vi "数据表比对.vi"(8 "error in (no error)":errorcluster, 9 "查询元素输入":string(combo), 10 "仪器日志参数":string, 11 "table输入":string(combo)) -> (0 "error out":errorcluster, 1 "columns输出":string[](array[string]), 2 "待发送第一条数据":string[](array[string]), 3 "待发送数据":string[][](table))   [LabVIEW 2016, in "数据传输系统.lvlib"]
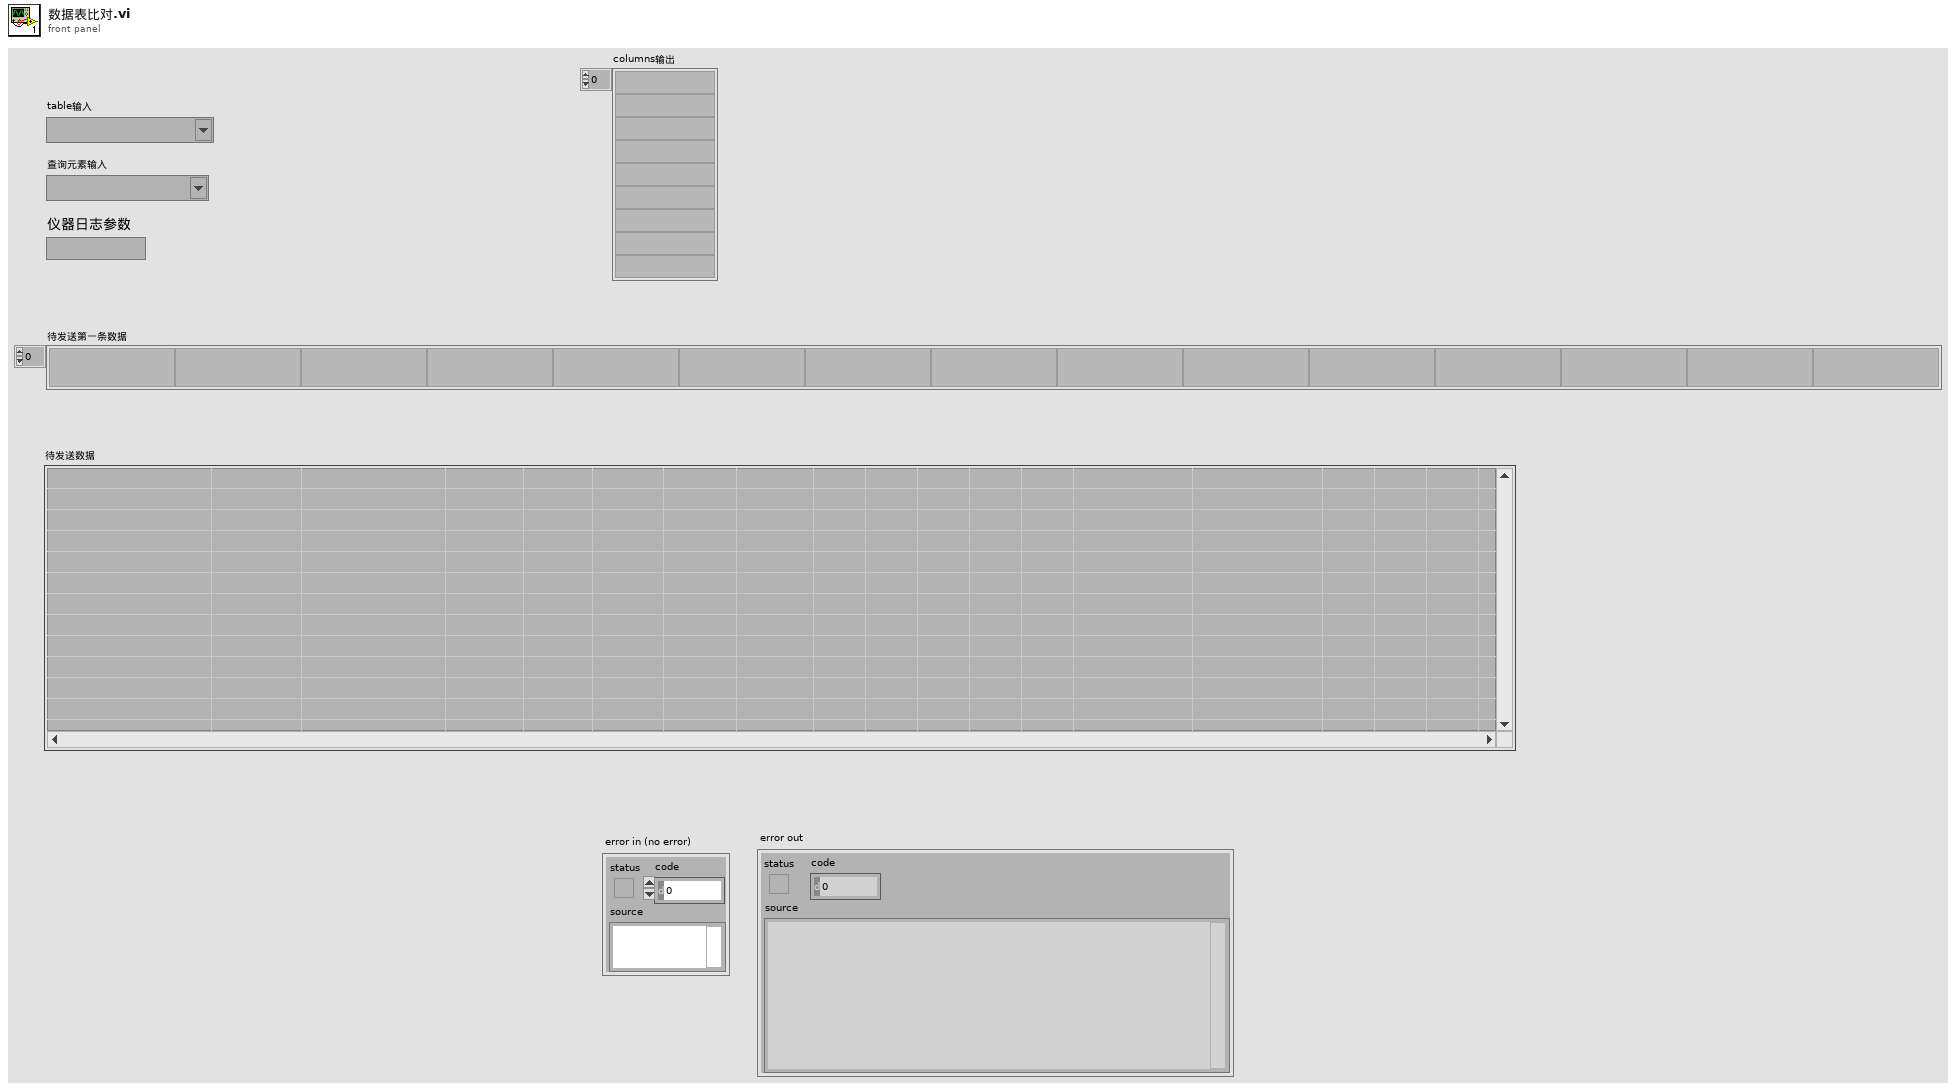
[diagram p1: front panel]
types:
  T1 = cluster{"氨氮仪器日志索引起始时间":string, "总磷仪器日志索引起始时间":string, "总氮仪器日志索引起始时间":string, "CODMn仪器日志索引起始时间":string, "CODCr仪器日志索引起始时间":string, "系统仪器日志索引起始时间":string, "氟化物仪器日志索引起始时间":string, "挥发酚仪器日志索引起始时间":string}
  T2 = cluster{"氨氮仪器参数索引起始时间":string, "总磷仪器参数索引起始时间":string, "总氮仪器参数索引起始时间":string, "CODMn仪器参数索引起始时间":string, "CODCr仪器参数索引起始时间":string, "DO仪器参数索引起始时间":string, "PH仪器参数索引起始时间":string, "比电导率仪器参数索引起始时间":string, "水温仪器参数索引起始时间":string, "浊度仪器参数索引起始时间":string, "叶绿素a仪器参数索引起始时间":string, "藻密度仪器参数索引起始时间":string, "ORP仪器参数索引起始时间":string, "氟化物仪器参数索引起始时间":string, "挥发酚仪器参数索引起始时间":string}
  T3 = typedef "数据传输系统.lvlib/应用环境.ctl" = enum16{"STD", "GB212", "婉仪平台"}
  T4 = cluster{"氨氮报警信息索引起始时间":string, "总磷报警信息索引起始时间":string, "总氮报警信息索引起始时间":string, "CODMn报警信息索引起始时间":string, "CODCr报警信息索引起始时间":string, "DO报警信息索引起始时间":string, "PH报警信息索引起始时间":string, "比电导率报警信息索引起始时间":string, "水温报警信息索引起始时间":string, "浊度报警信息索引起始时间":string, "叶绿素报警信息索引起始时间":string, "系统报警信息索引起始时间":string, "氟化物报警信息索引起始时间":string, "挥发酚报警信息索引起始时间":string}
  T5 = cluster{"氨氮零点核查索引起始时间":string, "总磷零点核查索引起始时间":string, "总氮零点核查索引起始时间":string, "CODMn零点核查索引起始时间":string, "CODCr零点核查索引起始时间":string, "亚硝酸盐零点核查索引起始时间":string, "硫化物零点核查索引起始时间":string, "ORP零点核查索引起始时间":string, "氟化物零点核查索引起始时间":string, "挥发酚零点核查索引起始时间":string}
  T6 = cluster{"氨氮标样核查索引起始时间":string, "总磷标样核查索引起始时间":string, "总氮标样核查索引起始时间":string, "CODMn标样核查索引起始时间":string, "CODCr标样核查索引起始时间":string, "DO标样核查索引起始时间":string, "PH标样核查索引起始时间":string, "比电导率标样核查索引起始时间":string, "水温标样核查索引起始时间":string, "浊度标样核查索引起始时间":string, "叶绿素a标样核查索引起始时间":string, "藻密度标样核查索引起始时间":string, "亚硝酸盐标样核查索引起始时间":string, "硫化物标样核查索引起始时间":string, "ORP标样核查索引起始时间":string, "氟化物标样核查索引起始时间":string, "挥发酚标样核查索引起始时间":string, "氯化物标样核查索引起始时间":string}
  T7 = cluster{"氨氮跨度核查索引起始时间":string, "总磷跨度核查索引起始时间":string, "总氮跨度核查索引起始时间":string, "CODMn跨度核查索引起始时间":string, "CODCr跨度核查索引起始时间":string, "亚硝酸盐跨度核查索引起始时间":string, "硫化物跨度核查索引起始时间":string, "ORP跨度核查索引起始时间":string, "氟化物跨度核查索引起始时间":string, "挥发酚跨度核查索引起始时间":string}
  T8 = typedef "LVDateTimeRec.ctl" = cluster{"秒数的小数部分":dbl, "秒":i32, "分":i32, "时":i32, "日":i32, "月":i32, "年":i32, "天数（周）":i32, "天数（年）":i32, "DST":i32}
  T9 = cluster{"氨氮加标回收索引起始时间":string, "总磷加标回收索引起始时间":string, "总氮加标回收索引起始时间":string, "CODMn加标回收索引起始时间":string, "CODCr加标回收索引起始时间":string, "氟化物加标回收索引起始时间":string, "挥发酚加标回收索引起始时间":string}
  T10 = cluster{"氨氮平行样索引起始时间":string, "总磷平行样索引起始时间":string, "总氮平行样索引起始时间":string, "CODMn平行样索引起始时间":string, "CODCr平行样索引起始时间":string, "氟化物平行样索引起始时间":string, "挥发酚平行样索引起始时间":string}
  T11 = cluster{"氨氮集成干预索引起始时间":string, "总磷集成干预索引起始时间":string, "总氮集成干预索引起始时间":string, "CODMn集成干预索引起始时间":string, "CODCr集成干预索引起始时间":string, "DO集成干预索引起始时间":string, "PH集成干预索引起始时间":string, "比电导率集成干预索引起始时间":string, "水温集成干预索引起始时间":string, "浊度集成干预索引起始时间":string, "叶绿素a集成干预索引起始时间":string, "藻密度集成干预索引起始时间":string, "亚硝酸盐集成干预索引起始时间":string, "硫化物集成干预索引起始时间":string, "ORP集成干预索引起始时间":string, "氟化物集成干预索引起始时间":string, "挥发酚集成干预索引起始时间":string, "氯化物集成干预索引起始时间":string}
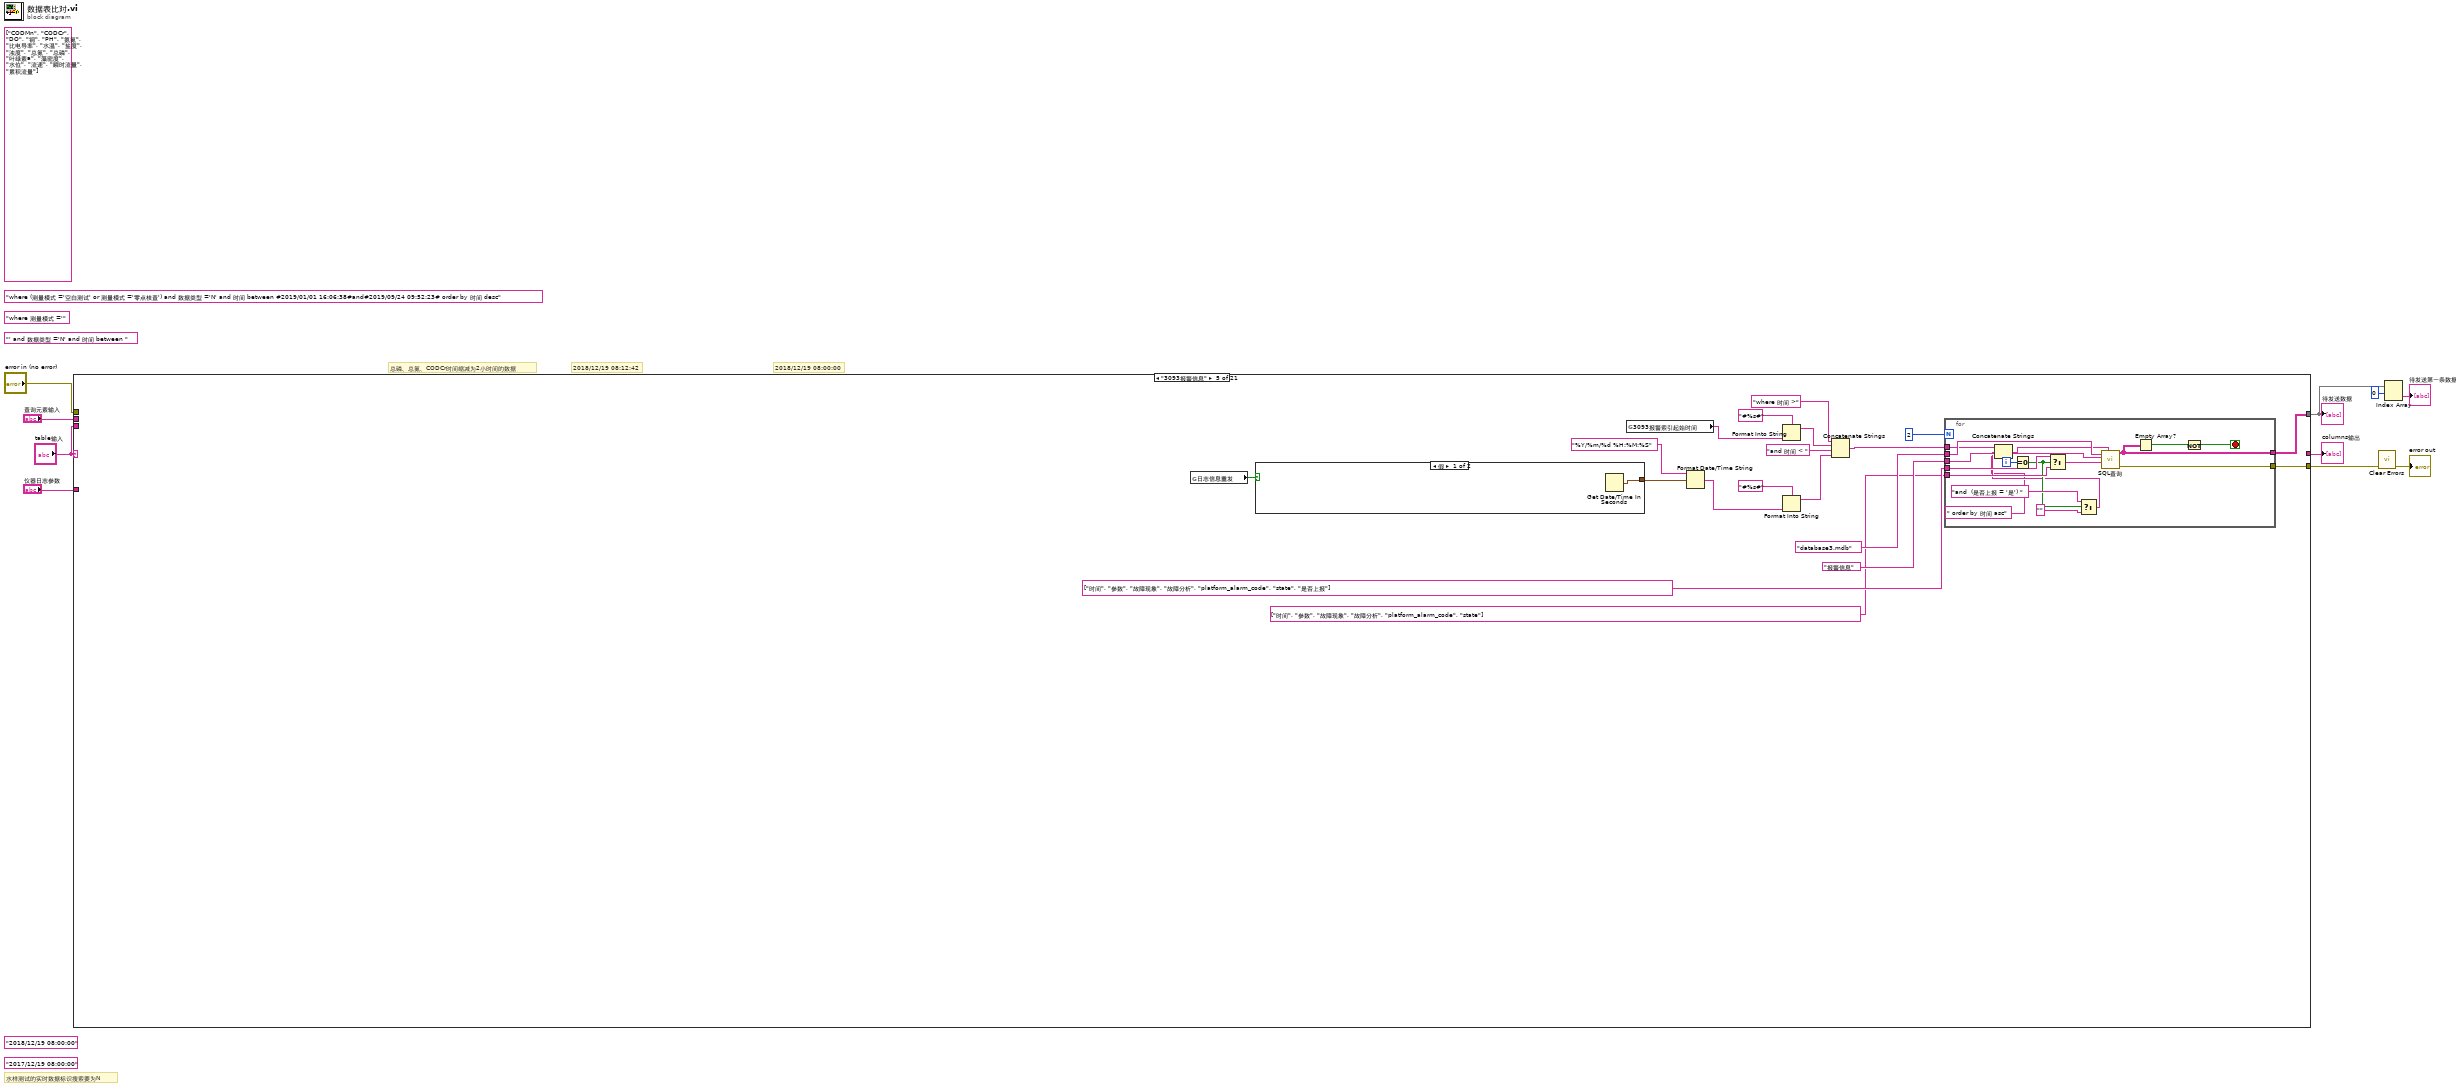
[diagram p0: block diagram]
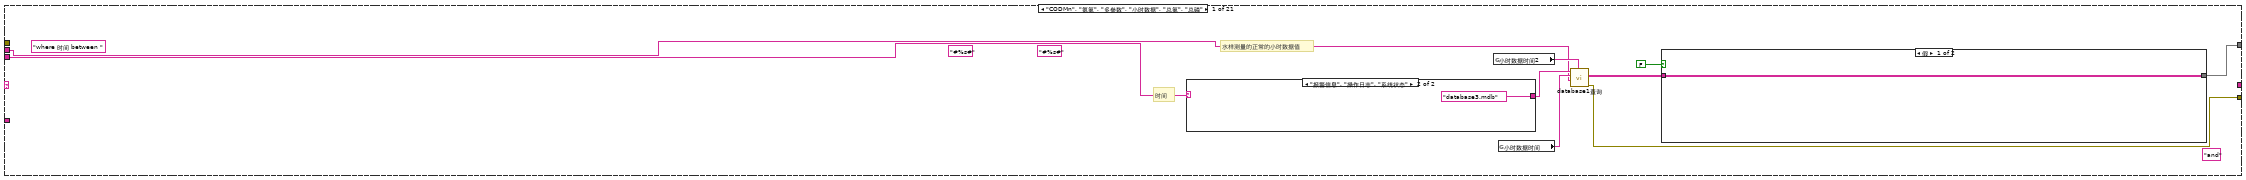
[diagram p2: hidden frame]
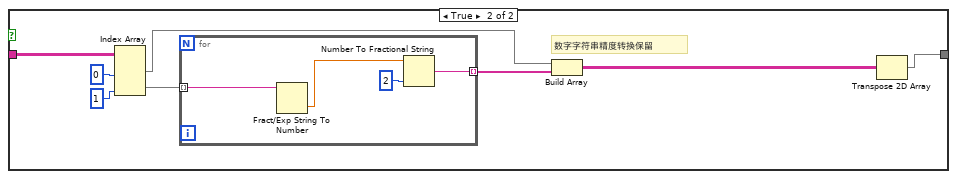
[diagram p3: hidden frame]
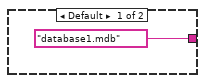
[diagram p4: hidden frame]
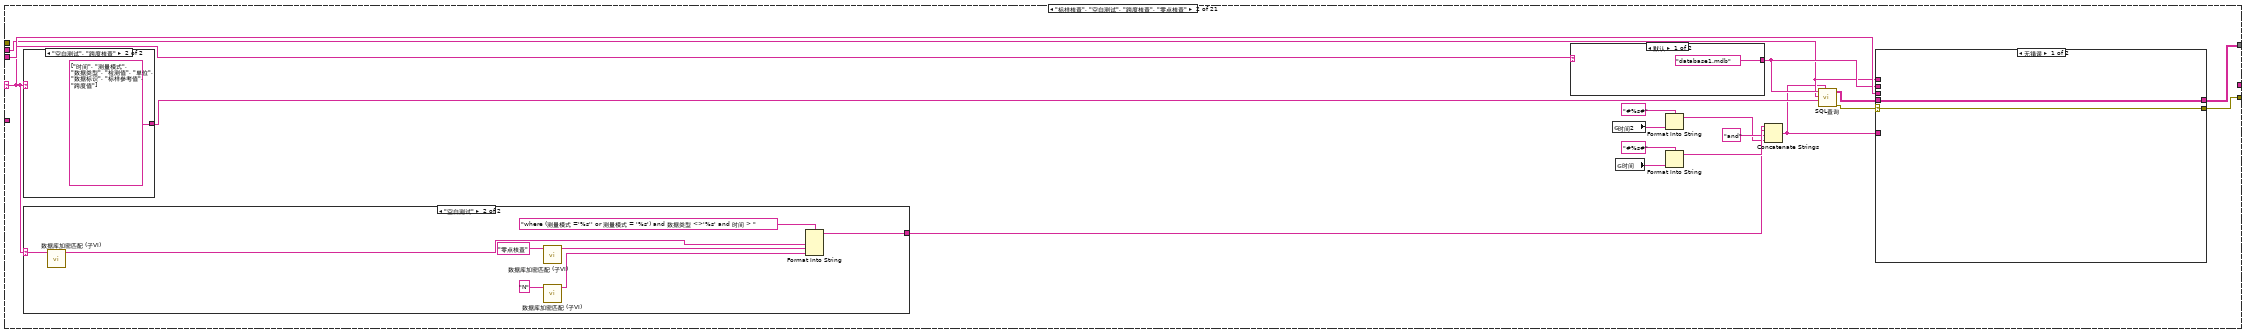
[diagram p5: hidden frame]
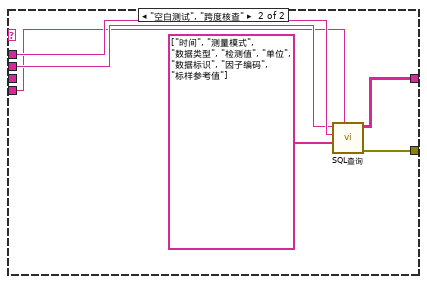
[diagram p7: hidden frame]
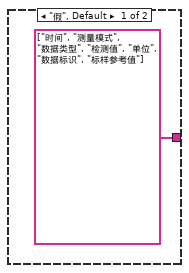
[diagram p8: hidden frame]
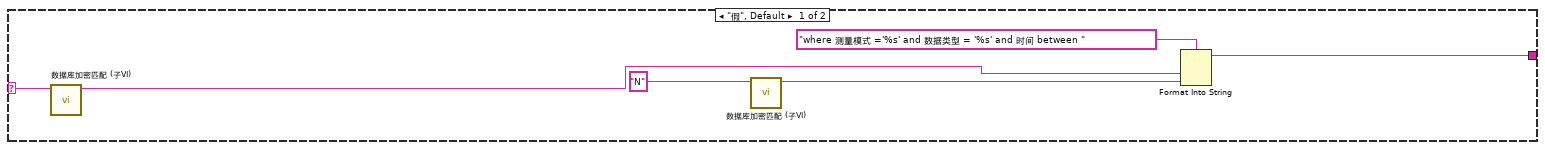
[diagram p9: hidden frame]
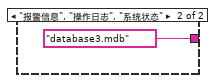
[diagram p10: hidden frame]
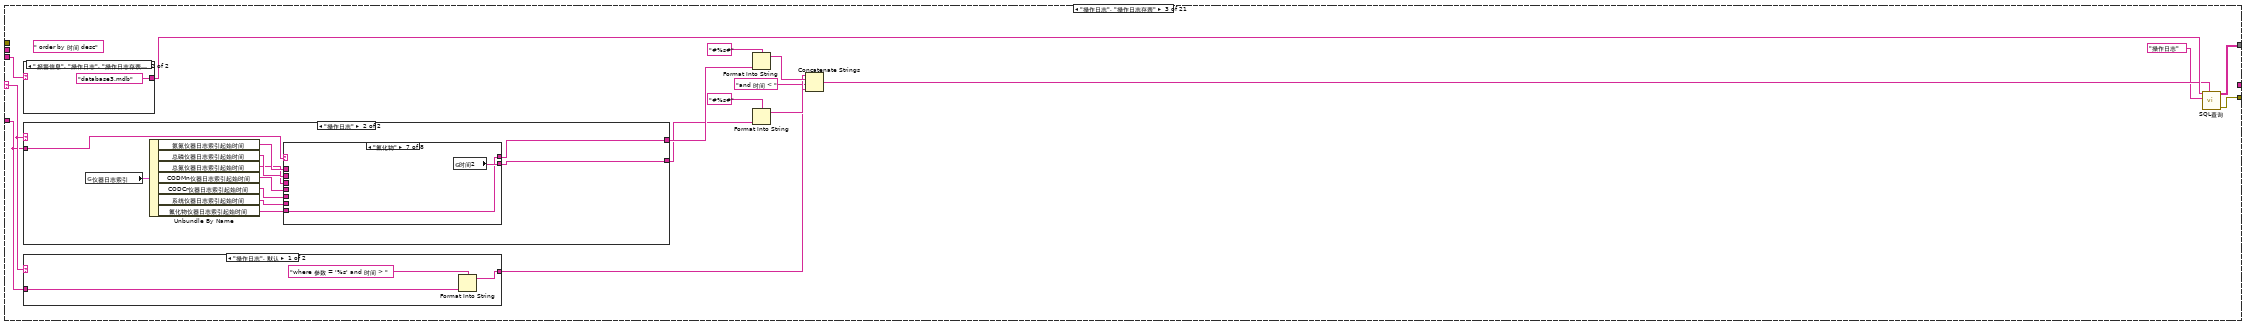
[diagram p11: hidden frame]
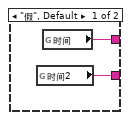
[diagram p12: hidden frame]
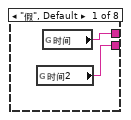
[diagram p13: hidden frame]
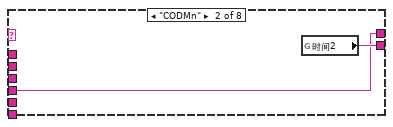
[diagram p14: hidden frame]
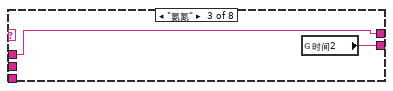
[diagram p15: hidden frame]
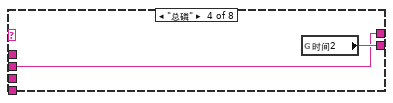
[diagram p16: hidden frame]
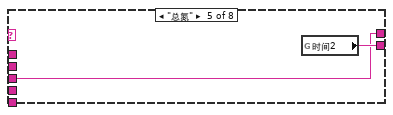
[diagram p17: hidden frame]
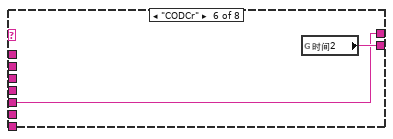
[diagram p18: hidden frame]
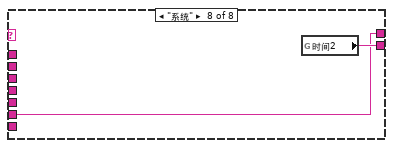
[diagram p19: hidden frame]
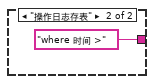
[diagram p20: hidden frame]
diagram:
  (unwired) "' and 数据类型 ='N' and 时间 between "
  (unwired) "where 测量模式 ='" ("condition")
  (unwired) "where (测量模式 ='空白测试' or 测量模式 ='零点核查') and 数据类型 ='N' and 时间 between #2019/01/01 16:06:38#and#2019/09/24 09:52:23# order by 时间 desc" ("condition")
  (unwired) string[] ["CODMn", "CODCr", "DO", "铜", "PH", "氨氮", "比电导率", "水温", "盐度", "浊度", "总氮", "总磷", "叶绿素a", "藻密度", "水位", "流速", "瞬时流量", "累积流量"] ("查询参数数组")
  (unwired) "2017/12/19 08:00:00"
  (unwired) "2018/12/19 08:00:00"
  # "水样测试的实时数据标识搜索要为N"
  # "2018/12/19 08:00:00"
  # "总磷、总氮、CODCr时间缩减为2小时间的数据"
  # "2018/12/19 08:12:42"
  n1 = case shown="\"3093报警信息\"" "table输入" {
    selector: "table输入" -> [_ w41 w91 _ _ _ _ _ _ w407 _ _ _ _ _ _ _ _ _ _ _]
    tunnel: "error in (no error)" -> [_ _ _ _ _ _ _ _ _ _ _ _ w535 _ _ _ _ _ _ _ _]
    tunnel: [w17 w35 w100 w153 w174 w210 w219 w278 w382 w421 w513 w532 w535 w536 w735 w782 w849 w920 w962 w1005 w1056] -> w8
    tunnel: [w13 w36 w98 w151 w172 w208 w246 w280 w374 w419 w497 w531 w533 w538 w733 w785 w847 w923 w965 w1008 w1058] -> w1
    tunnel: "table输入" -> [w19 w52 w102 _ _ _ w218 w281 _ w411 _ w528 _ _ _ _ _ _ _ _ _]
    tunnel: "查询元素输入" -> [w11 w39 _ _ _ _ _ _ _ _ _ _ _ w542 w720 w767 w835 w912 w954 w995 w1052]
    tunnel: "仪器日志参数" -> [_ _ w88 _ _ w196 w213 w269 w353 w406 w496 _ _ _ _ _ _ _ _ _ _]
    tunnel: [_ _ _ _ _ _ _ _ _ _ _ w527 _ _ _ _ _ _ _ _ _] -> w2
    frame "CODMn", "氨氮", "多参数", "小时数据", "总氮", "总磷" {
      (unwired) "and" ("字符串")
      (unwired) "#%s#" ("初始字符串")
      (unwired) "#%s#" ("初始字符串")
      (unwired) "where 时间 between " ("condition")
      # "水样测量的正常的小时数据值"
      # "时间"
      n2 = case shown="\"报警信息\", \"操作日志\", \"系统状态\"" w19 {
        tunnel: ["database1.mdb" ("database") "database3.mdb" ("database")] -> w18
        frame Default {
        }
        frame "报警信息", "操作日志", "系统状态" {
        }
      }
      n3 = global read "全局 时间2.vi" "小时数据时间2"() -> (w15:string)
      n4 = global read "全局 水样时间.vi" "小时数据时间"() -> (w16:string)
      n5 = call "database1查询.vi"("时间2"=w15, "table"=w11, "时间1"=w16, "database"=w18) -> ("error out"=w17:errorcluster, "data"=w14:string[][])  [unwired: 3 in, 2 out]
      n6 = case shown="假" FALSE {
        tunnel: w14 -> [w20 w28]
        tunnel: [w20 w21] -> w13
        frame False {
        }
        frame True {
          # "数字字符串精度转换保留"
          n7 = Index Array(array=w28, index (col) #1=0 ("禁用的索引 (列)"), index (col) #2=1 ("索引 (列)")) -> (element #1=w24:string[], element #2=w25:string[])  [unwired: 2 in]
          n8 = for {
            tunnel: w25 -> [w30] mode=indexing
            tunnel: [w29] -> w23 mode=indexing
            n9 = Fract/Exp String To Number(string=w30) -> (number=w31:dbl)  [unwired: 3 in, 1 out]
            n10 = Number To Fractional String(number=w31, precision (6)=i16 2 ("精度(6)")) -> (F-format string=w29:string)  [unwired: 2 in]
          }
          n11 = Build Array(w24, w23) -> (w22:string[][])
          n12 = Transpose 2D Array(2D array=w22) -> (transposed array=w21:string[][])
        }
      }
    }
    frame "标样核查", "空白测试", "跨度核查", "零点核查" {
      n13 = case shown="\"空白测试\", \"跨度核查\"" w41 {
        tunnel: [string[] ["时间", "测量模式", "数据类型", "检测值", "单位", "数据标识", "标样参考值"] ("columns") string[] ["时间", "测量模式", "数据类型", "检测值", "单位", "数据标识", "标样参考值", "跨度值"] ("columns")] -> w43
        frame "假", Default {
        }
        frame "空白测试", "跨度核查" {
        }
      }
      n14 = case shown="\"空白测试\"" w41 {
        selector: w41 -> [w74 w81]
        tunnel: [w75 w83] -> w44
        frame "假", Default {
          n15 = call "数据库加密匹配 (子VI).vi"("输入参数"=w74) -> ("Encoded String"=w73:string)  [unwired: 10 in]
          n16 = call "数据库加密匹配 (子VI).vi"("输入参数"="N" ("字符串")) -> ("Encoded String"=w71:string)  [unwired: 10 in]
          n17 = Format Into String(format string="where 测量模式 ='%s' and 数据类型 = '%s' and 时间 between " ("格式字符串"), w73, w71) -> (resulting string=w75:string)  [unwired: 2 in, 1 out]
        }
        frame "空白测试" {
          n18 = call "数据库加密匹配 (子VI).vi"("输入参数"=w81) -> ("Encoded String"=w82:string)  [unwired: 10 in]
          n19 = call "数据库加密匹配 (子VI).vi"("输入参数"="零点核查") -> ("Encoded String"=w79:string)  [unwired: 10 in]
          n20 = call "数据库加密匹配 (子VI).vi"("输入参数"="N") -> ("Encoded String"=w77:string)  [unwired: 10 in]
          n21 = Format Into String(format string="where (测量模式 ='%s'' or 测量模式 = '%s') and 数据类型 <>'%s' and 时间 > " ("格式字符串"), w82, w79, w77) -> (resulting string=w83:string)  [unwired: 2 in, 1 out]
        }
      }
      n22 = case shown="默认" w52 {
        tunnel: ["database1.mdb" ("database") "database3.mdb" ("database")] -> w40
        frame Default {
        }
        frame "报警信息", "操作日志", "系统状态" {
        }
      }
      n23 = global read "全局 时间2.vi" "时间2"() -> (w45:string)
      n24 = global read "全局 水样时间.vi" "时间"() -> (w46:string)
      n25 = Format Into String(format string="#%s#" ("初始字符串"), w45) -> (resulting string=w47:string)  [unwired: 2 in, 1 out]
      n26 = Format Into String(format string="#%s#" ("初始字符串"), w46) -> (resulting string=w51:string)  [unwired: 2 in, 1 out]
      n27 = Concatenate Strings(w44, w51, "and" ("字符串"), w47) -> (w38:string)
      n28 = call "SQL查询.vi"("condition"=w38, "columns"=w43, "table输入"=w39, "database"=w40) -> ("error out"=w42:errorcluster, "data"=w37:string[][])  [unwired: 4 in, 2 out]
      n29 = case shown="无错误" w42 {
        selector: w42 -> [w53 _]
        tunnel: w41 -> [_ w61]
        tunnel: w39 -> [_ w60]
        tunnel: w40 -> [_ w59]
        tunnel: w38 -> [_ w58]
        tunnel: w37 -> [w54 w56]
        tunnel: [w54 w57] -> w36
        tunnel: [w53 w55] -> w35
        frame No Error {
        }
        frame Error {
          # "兼容旧数据库没有跨度值版本"
          n30 = case shown="\"假\", 默认" w61 {
            tunnel: w60 -> [_ w67]
            tunnel: w59 -> [_ w66]
            tunnel: w58 -> [_ w65]
            tunnel: [w62 w64] -> w57
            tunnel: w56 -> [w62 _]
            tunnel: [_ w63] -> w55
            frame "假", Default {
            }
            frame "空白测试", "跨度核查" {
              n31 = call "SQL查询.vi"("condition"=w65, "columns"=string[] ["时间", "测量模式", "数据类型", "检测值", "单位", "数据标识", "因子编码", "标样参考值"], "table输入"=w67, "database"=w66) -> ("error out"=w63:errorcluster, "data"=w64:string[][])  [unwired: 4 in, 2 out]
            }
          }
        }
      }
    }
    frame "操作日志", "操作日志存表" {
      (unwired) " order by 时间 desc" ("字符串")
      n32 = case shown="\"报警信息\", \"操作日志\", \"操作日志存表\", \"系统状态\"" w102 {
        tunnel: ["database1.mdb" ("database") "database3.mdb" ("database")] -> w101
        frame Default {
        }
        frame "报警信息", "操作日志", "操作日志存表", "系统状态" {
        }
      }
      n33 = case shown="\"操作日志\"" w91 {
        tunnel: [w104 w114] -> w90
        tunnel: [w103 w106] -> w89
        tunnel: w88 -> [_ w115]
        frame "假", Default {
          n34 = global read "全局 时间2.vi" "时间2"() -> (w103:string)
          n35 = global read "全局 水样时间.vi" "时间"() -> (w104:string)
        }
        frame "操作日志" {
          n36 = global read "全局 时间2.vi" "仪器日志索引"() -> (w113:T1)
          n37 = Unbundle By Name(w113) -> ("氨氮仪器日志索引起始时间"=w112:string, "总磷仪器日志索引起始时间"=w111:string, "总氮仪器日志索引起始时间"=w110:string, "CODMn仪器日志索引起始时间"=w109:string, "CODCr仪器日志索引起始时间"=w108:string, "系统仪器日志索引起始时间"=w107:string, "氟化物仪器日志索引起始时间"=w105:string)
          n38 = case shown="\"氟化物\"" w115 {
            tunnel: [w116 w119 w121 w123 w125 w127 w129 w131] -> w106
            tunnel: [w117 w118 w120 w122 w124 w126 w128 w130] -> w114
            tunnel: w112 -> [_ _ w120 _ _ _ _ _]
            tunnel: w111 -> [_ _ _ w122 _ _ _ _]
            tunnel: w110 -> [_ _ _ _ w124 _ _ _]
            tunnel: w109 -> [_ w118 _ _ _ _ _ _]
            tunnel: w108 -> [_ _ _ _ _ w126 _ _]
            tunnel: w107 -> [_ _ _ _ _ _ _ w130]
            tunnel: w105 -> [_ _ _ _ _ _ w128 _]
            frame "假", Default {
              n39 = global read "全局 时间2.vi" "时间2"() -> (w116:string)
              n40 = global read "全局 水样时间.vi" "时间"() -> (w117:string)
            }
            frame "CODMn" {
              n41 = global read "全局 时间2.vi" "时间2"() -> (w119:string)
            }
            frame "氨氮" {
              n42 = global read "全局 时间2.vi" "时间2"() -> (w121:string)
            }
            frame "总磷" {
              n43 = global read "全局 时间2.vi" "时间2"() -> (w123:string)
            }
            frame "总氮" {
              n44 = global read "全局 时间2.vi" "时间2"() -> (w125:string)
            }
            frame "CODCr" {
              n45 = global read "全局 时间2.vi" "时间2"() -> (w127:string)
            }
            frame "氟化物" {
              n46 = global read "全局 时间2.vi" "时间2"() -> (w129:string)
            }
            frame "系统" {
              n47 = global read "全局 时间2.vi" "时间2"() -> (w131:string)
            }
          }
        }
      }
      n48 = case shown="\"操作日志\", 默认" w91 {
        tunnel: [w133 "where 时间 >" ("condition")] -> w93
        tunnel: w88 -> [w132 _]
        frame "操作日志", Default {
          n49 = Format Into String(format string="where 参数 = '%s' and 时间 > " ("condition"), w132) -> (resulting string=w133:string)  [unwired: 2 in, 1 out]
        }
        frame "操作日志存表" {
        }
      }
      n50 = Format Into String(format string="#%s#" ("初始字符串"), w90) -> (resulting string=w97:string)  [unwired: 2 in, 1 out]
      n51 = Format Into String(format string="#%s#" ("初始字符串"), w89) -> (resulting string=w94:string)  [unwired: 2 in, 1 out]
      n52 = Concatenate Strings(w93, w97, "and 时间 < " ("字符串"), w94) -> (w99:string)
      n53 = call "SQL查询.vi"("condition"=w99, "table输入"="操作日志", "database"=w101) -> ("error out"=w100:errorcluster, "data"=w98:string[][])  [unwired: 5 in, 2 out]
    }
    frame "3092日志信息" {
      n54 = global read "断电保存全局.vi" "日志信息重发"() -> (w138:bool)
      n55 = case shown="真" w138 {
        tunnel: [w155 w156] -> w141
        frame False {
          n56 = Get Date/Time In Seconds() -> (seconds since 1Jan1904=w155:timestamp)
        }
        frame True {
          n57 = global read "断电保存全局.vi" "数据重发结束时间"() -> (w156:timestamp)
        }
      }
      n58 = global read "全局 时间2.vi" "3092日志索引起始时间"() -> (w143:string)
      n59 = Format Date/Time String(time format string (%c)="%Y/%m/%d %H:%M:%S" ("时间格式字符串(%c)"), seconds (now)=w141) -> (date/time string=w140:string)  [unwired: 1 in]
      n60 = Format Into String(format string="#%s#" ("初始字符串"), w143) -> (resulting string=w150:string)  [unwired: 2 in, 1 out]
      n61 = Format Into String(format string="#%s#" ("初始字符串"), w140) -> (resulting string=w147:string)  [unwired: 2 in, 1 out]
      n62 = Concatenate Strings("where 时间 >" ("condition"), w150, "and 时间 < " ("字符串"), w147, " order by 时间 asc" ("字符串")) -> (w152:string)
      n63 = call "SQL查询.vi"("condition"=w152, "table输入"="操作日志", "database"="database3.mdb") -> ("error out"=w153:errorcluster, "data"=w151:string[][])  [unwired: 5 in, 2 out]
    }
    frame "3093报警信息" {
      n64 = global read "断电保存全局.vi" "日志信息重发"() -> (w161:bool)
      n65 = case shown="假" w161 {
        tunnel: [w193 w194] -> w160
        frame False {
          n66 = Get Date/Time In Seconds() -> (seconds since 1Jan1904=w193:timestamp)
        }
        frame True {
          n67 = global read "断电保存全局.vi" "数据重发结束时间"() -> (w194:timestamp)
        }
      }
      n68 = global read "全局 时间2.vi" "3093报警索引起始时间"() -> (w164:string)
      n69 = Format Date/Time String(time format string (%c)="%Y/%m/%d %H:%M:%S" ("时间格式字符串(%c)"), seconds (now)=w160) -> (date/time string=w162:string)  [unwired: 1 in]
      n70 = Format Into String(format string="#%s#" ("初始字符串"), w164) -> (resulting string=w171:string)  [unwired: 2 in, 1 out]
      n71 = Format Into String(format string="#%s#" ("初始字符串"), w162) -> (resulting string=w168:string)  [unwired: 2 in, 1 out]
      n72 = Concatenate Strings("where 时间 >" ("condition"), w171, "and 时间 < " ("字符串"), w168) -> (w173:string)
      n73 = for {
        N: 2 -> [_]
        tunnel: "database3.mdb" ("database") -> [w192]
        tunnel: [w191] -> w174
        tunnel: w173 -> [w182]
        tunnel: [w189] -> w172
        tunnel: "报警信息" ("table输入") -> [w190]
        tunnel: string[] ["时间", "参数", "故障现象", "故障分析", "platform_alarm_code", "state", "是否上报"] ("columns") -> [w185]
        tunnel: string[] ["时间", "参数", "故障现象", "故障分析", "platform_alarm_code", "state"] ("columns") -> [w184]
        i -> [w186]
        stop <- w187 stop-if-true
        n74 = Equal To 0?(x=w186) -> (x = 0?=w179:bool)
        n75 = Select(t=w185, s=w179, f=w184) -> (s? t:f=w183:string[])
        n76 = Select(t="and  (是否上报 = '是') " ("字符串"), s=w179, f="") -> (s? t:f=w177:string)
        n77 = Concatenate Strings(w182, w177, " order by 时间 asc" ("字符串")) -> (w181:string)
        n78 = call "SQL查询.vi"("condition"=w181, "columns"=w183, "table输入"=w190, "database"=w192) -> ("error out"=w191:errorcluster, "data"=w189:string[][])  [unwired: 4 in, 2 out]
        n79 = Empty Array?(array=w189) -> (empty?=w188:bool)
        n80 = Not(x=w188) -> (.not. x?=w187:bool)
      }
    }
    frame "提取操作日志" {
      n81 = call "数据库加密匹配 (子VI).vi"("输入参数"=w196) -> ("Encoded String"=w195:string)  [unwired: 10 in]
      n82 = global read "全局 时间2.vi" "时间2"() -> (w199:string)
      n83 = global read "全局 水样时间.vi" "时间"() -> (w200:string)
      n84 = Format Into String(format string="where 参数 = '%s' and 时间 between" ("condition"), w195) -> (resulting string=w202:string)  [unwired: 2 in, 1 out]
      n85 = Format Into String(format string="#%s#" ("初始字符串"), w200) -> (resulting string=w207:string)  [unwired: 2 in, 1 out]
      n86 = Format Into String(format string="#%s#" ("初始字符串"), w199) -> (resulting string=w203:string)  [unwired: 2 in, 1 out]
      n87 = Concatenate Strings(w202, w207, "and" ("字符串"), w203) -> (w209:string)
      n88 = call "SQL查询.vi"("condition"=w209, "table输入"="操作日志", "database"="database3.mdb") -> ("error out"=w210:errorcluster, "data"=w208:string[][])  [unwired: 5 in, 2 out]
    }
    frame "3090仪器参数" {
      (unwired) string[] ["时间", "参数", "测量量程", "测量精度", "测量间隔", "消解温度", "消解时长", "空白校准时间", "曲线截距", "曲线斜率", "测量检出限", "测量信号值", "线性相关系数", "二次多项式系数", "标样校准时间", "稀释倍数", "三项式系数", "空白标定系数", "量程系数", "F0/ORPA", "F1/ORPB", "F2/ORPK", "F3", "F4", "F5", "F6", "F7", "X0/滴定数", "量程"] ("columns输出")
      n89 = case shown="\"3090仪器参数\"" w218 {
        tunnel: [w249 w250] -> w234
        frame "3090仪器参数" {
          n90 = global read "全局 时间2.vi" "3090仪器参数索引"() -> (w249:T2)
        }
        frame "仪器参数", Default {
          n91 = global read "全局 时间2.vi" "仪器参数索引"() -> (w250:T2)
        }
      }
      n92 = call "数据库加密匹配 (子VI).vi"("输入参数"=w213) -> ("Encoded String"=w212:string)  [unwired: 10 in]
      n93 = global read "断电保存全局.vi" "数据发送延时时间/s"() -> (w215:i32)
      n94 = Unbundle By Name(w234) -> ("氨氮仪器参数索引起始时间"=w233:string, "总磷仪器参数索引起始时间"=w232:string, "总氮仪器参数索引起始时间"=w231:string, "CODMn仪器参数索引起始时间"=w230:string, "CODCr仪器参数索引起始时间"=w229:string, "DO仪器参数索引起始时间"=w227:string, "PH仪器参数索引起始时间"=w226:string, "比电导率仪器参数索引起始时间"=w225:string, "水温仪器参数索引起始时间"=w224:string, "浊度仪器参数索引起始时间"=w223:string, "叶绿素a仪器参数索引起始时间"=w222:string, "藻密度仪器参数索引起始时间"=w221:string, "ORP仪器参数索引起始时间"=w220:string, "氟化物仪器参数索引起始时间"=w211:string)
      n95 = Format Into String(format string="where 参数 = '%s' and 时间 > " ("condition"), w212) -> (resulting string=w241:string)  [unwired: 2 in, 1 out]
      n96 = Get Date/Time In Seconds() -> (seconds since 1Jan1904=w216:timestamp)
      n97 = case shown="\"氟化物\"" w213 {
        tunnel: w233 -> [_ _ w253 _ _ _ _ _ _ _ _ _ _ _ _]
        tunnel: w232 -> [_ _ _ w254 _ _ _ _ _ _ _ _ _ _ _]
        tunnel: w231 -> [_ _ _ _ w255 _ _ _ _ _ _ _ _ _ _]
        tunnel: w230 -> [w251 w252 _ _ _ _ _ _ _ _ _ _ _ _ _]
        tunnel: w229 -> [_ _ _ _ _ w256 _ _ _ _ _ _ _ _ _]
        tunnel: [w251 w252 w253 w254 w255 w256 w257 w258 w259 w260 w261 w262 w263 w264 w265] -> w228
        tunnel: w227 -> [_ _ _ _ _ _ w257 _ _ _ _ _ _ _ _]
        tunnel: w226 -> [_ _ _ _ _ _ _ w258 _ _ _ _ _ _ _]
        tunnel: w225 -> [_ _ _ _ _ _ _ _ w259 _ _ _ _ _ _]
        tunnel: w224 -> [_ _ _ _ _ _ _ _ _ w260 _ _ _ _ _]
        tunnel: w223 -> [_ _ _ _ _ _ _ _ _ _ w261 _ _ _ _]
        tunnel: w222 -> [_ _ _ _ _ _ _ _ _ _ _ w262 _ _ _]
        tunnel: w221 -> [_ _ _ _ _ _ _ _ _ _ _ _ w263 _ _]
        tunnel: w220 -> [_ _ _ _ _ _ _ _ _ _ _ _ _ w264 _]
        tunnel: w211 -> [_ _ _ _ _ _ _ _ _ _ _ _ _ _ w265]
        frame "假", Default {
        }
        frame "CODMn" {
        }
        frame "氨氮" {
        }
        frame "总磷" {
        }
        frame "总氮" {
        }
        frame "CODCr" {
        }
        frame "溶解氧" {
        }
        frame "PH" {
        }
        frame "电导率" {
        }
        frame "水温" {
        }
        frame "浊度" {
        }
        frame "叶绿素" {
        }
        frame "藻密度" {
        }
        frame "ORP" {
        }
        frame "氟化物" {
        }
      }
      n98 = Subtract(x=w216, y=w215) -> (x-y=w214:timestamp)
      n99 = Format Date/Time String(time format string (%c)="%Y/%m/%d %H:%M:%S" ("时间格式字符串(%c)"), seconds (now)=w214) -> (date/time string=w237:string)  [unwired: 1 in]
      n100 = Search and Replace String(input string=w237, search string="." ("搜索字符串")) -> (result string=w235:string)  [unwired: 6 in, 3 out]
      n101 = Format Into String(format string="#%s#" ("初始字符串"), w235) -> (resulting string=w242:string)  [unwired: 2 in, 1 out]
      n102 = Format Into String(format string="#%s#" ("初始字符串"), w228) -> (resulting string=w245:string)  [unwired: 2 in, 1 out]
      n103 = Concatenate Strings(w241, w245, "and 时间 < " ("字符串"), w242, " order by 时间 asc" ("字符串")) -> (w247:string)
      n104 = call "SQL查询.vi"("condition"=w247, "table输入"=w218, "database"="database3.mdb") -> ("error out"=w219:errorcluster, "data"=w246:string[][])  [unwired: 5 in, 2 out]
    }
    frame "仪器参数" {
      n105 = case shown="\"仪器参数\", 默认" w281 {
        tunnel: [w336 w337] -> w298
        frame "3090仪器参数" {
          n106 = global read "全局 时间2.vi" "3090仪器参数索引"() -> (w336:T2)
        }
        frame "仪器参数", Default {
          n107 = global read "全局 时间2.vi" "仪器参数索引"() -> (w337:T2)
        }
      }
      n108 = global read "断电保存全局.vi" "应用环境"() -> (w271:T3)
      n109 = case shown="\"GB212\", 默认" w271 {
        tunnel: [w314 string[] ["时间", "数据类型", "测量量程", "测量精度", "测量间隔", "消解温度", "消解时长", "空白校准时间", "曲线截距", "曲线斜率", "测量检出限", "测量信号值", "线性相关系数", "二次多项式系数", "标样校准时间"] ("columns输出")] -> w284
        tunnel: w269 -> [w313 _]
        frame "STD" {
          n110 = case shown="\"CODMn\"" w313 {
            tunnel: [string[] ["时间", "数据类型", "测量量程", "测量精度", "测量间隔", "消解温度", "消解时长", "空白校准时间", "曲线截距", "曲线斜率", "测量检出限", "测量信号值", "线性相关系数", "二次多项式系数", "标样校准时间", "量程"] ("columns输出") string[] ["时间", "数据类型", "测量量程", "测量精度", "测量间隔", "消解温度", "消解时长", "空白校准时间", "曲线截距", "曲线斜率", "测量检出限", "测量信号值", "线性相关系数", "二次多项式系数", "标样校准时间", "量程标识"] ("columns输出")] -> w314
            frame "CODMn" {
            }
            frame "", Default {
            }
          }
        }
        frame "GB212", Default {
        }
      }
      n111 = Unbundle By Name(w298) -> ("氨氮仪器参数索引起始时间"=w297:string, "总磷仪器参数索引起始时间"=w296:string, "总氮仪器参数索引起始时间"=w295:string, "CODMn仪器参数索引起始时间"=w294:string, "CODCr仪器参数索引起始时间"=w293:string, "DO仪器参数索引起始时间"=w292:string, "PH仪器参数索引起始时间"=w291:string, "比电导率仪器参数索引起始时间"=w290:string, "水温仪器参数索引起始时间"=w289:string, "浊度仪器参数索引起始时间"=w288:string, "叶绿素a仪器参数索引起始时间"=w287:string, "藻密度仪器参数索引起始时间"=w286:string, "ORP仪器参数索引起始时间"=w285:string, "氟化物仪器参数索引起始时间"=w266:string)
      n112 = case shown="\"氟化物\"" w269 {
        tunnel: w297 -> [_ _ w340 _ _ _ _ _ _ _ _ _ _ _ _]
        tunnel: w296 -> [_ _ _ w341 _ _ _ _ _ _ _ _ _ _ _]
        tunnel: w295 -> [_ _ _ _ w342 _ _ _ _ _ _ _ _ _ _]
        tunnel: w294 -> [w338 w339 _ _ _ _ _ _ _ _ _ _ _ _ _]
        tunnel: w293 -> [_ _ _ _ _ w343 _ _ _ _ _ _ _ _ _]
        tunnel: [w338 w339 w340 w341 w342 w343 w344 w345 w346 w347 w348 w349 w350 w351 w352] -> w283
        tunnel: w292 -> [_ _ _ _ _ _ w344 _ _ _ _ _ _ _ _]
        tunnel: w291 -> [_ _ _ _ _ _ _ w345 _ _ _ _ _ _ _]
        tunnel: w290 -> [_ _ _ _ _ _ _ _ w346 _ _ _ _ _ _]
        tunnel: w289 -> [_ _ _ _ _ _ _ _ _ w347 _ _ _ _ _]
        tunnel: w288 -> [_ _ _ _ _ _ _ _ _ _ w348 _ _ _ _]
        tunnel: w287 -> [_ _ _ _ _ _ _ _ _ _ _ w349 _ _ _]
        tunnel: w286 -> [_ _ _ _ _ _ _ _ _ _ _ _ w350 _ _]
        tunnel: w285 -> [_ _ _ _ _ _ _ _ _ _ _ _ _ w351 _]
        tunnel: w266 -> [_ _ _ _ _ _ _ _ _ _ _ _ _ _ w352]
        frame "假", Default {
        }
        frame "CODMn" {
        }
        frame "氨氮" {
        }
        frame "总磷" {
        }
        frame "总氮" {
        }
        frame "CODCr" {
        }
        frame "溶解氧" {
        }
        frame "PH" {
        }
        frame "电导率" {
        }
        frame "水温" {
        }
        frame "浊度" {
        }
        frame "叶绿素" {
        }
        frame "藻密度" {
        }
        frame "ORP" {
        }
        frame "氟化物" {
        }
      }
      n113 = global read "断电保存全局.vi" "日志信息重发"() -> (w268:bool)
      n114 = case shown="假" w268 {
        tunnel: [w309 w312] -> w267
        frame False {
          n115 = global read "断电保存全局.vi" "数据发送延时时间/s"() -> (w310:i32)
          n116 = Get Date/Time In Seconds() -> (seconds since 1Jan1904=w311:timestamp)
          n117 = Subtract(x=w311, y=w310) -> (x-y=w309:timestamp)
        }
        frame True {
          n118 = global read "断电保存全局.vi" "数据重发结束时间"() -> (w312:timestamp)
        }
      }
      n119 = Format Into String(format string="#%s#" ("初始字符串"), w283) -> (resulting string=w306:string)  [unwired: 2 in, 1 out]
      n120 = call "数据库加密匹配 (子VI).vi"("输入参数"="N") -> ("Encoded String"=w272:string)  [unwired: 10 in]
      n121 = Format Date/Time String(time format string (%c)="%Y/%m/%d %H:%M:%S" ("时间格式字符串(%c)"), seconds (now)=w267) -> (date/time string=w300:string)  [unwired: 1 in]
      n122 = Search and Replace String(input string=w300, search string="." ("搜索字符串")) -> (result string=w282:string)  [unwired: 6 in, 3 out]
      n123 = Format Into String(format string="where 数据类型 = '%s' and 时间 > " ("condition"), w272) -> (resulting string=w274:string)  [unwired: 2 in, 1 out]
      n124 = Format Into String(format string="#%s#" ("初始字符串"), w282) -> (resulting string=w303:string)  [unwired: 2 in, 1 out]
      n125 = Concatenate Strings(w274, w306, "and 时间 < " ("字符串"), w303, " order by 时间 asc" ("字符串")) -> (w307:string)
      n126 = call "SQL查询.vi"("condition"=w307, "columns"=w284, "table输入"=w269, "database"="database1.mdb") -> ("error out"=w277:errorcluster, "data"=w279:string[][])  [unwired: 4 in, 2 out]
      n127 = Empty Array?(array=w279) -> ()  [unwired: 1 out]
      n128 = case shown="假" FALSE {
        tunnel: w269 -> [_ w333]
        tunnel: w283 -> [_ w329]
        tunnel: w282 -> [_ w325]
        tunnel: w281 -> [_ w322]
        tunnel: [w319 w321] -> w280
        tunnel: w279 -> [w319 _]
        tunnel: [w318 w320] -> w278
        tunnel: w277 -> [w318 _]
        frame False {
        }
        frame True {
          n129 = Format Into String(format string="#%s#" ("初始字符串"), w329) -> (resulting string=w328:string)  [unwired: 2 in, 1 out]
          n130 = Format Into String(format string="#%s#" ("初始字符串"), w325) -> (resulting string=w324:string)  [unwired: 2 in, 1 out]
          n131 = Format Into String(format string="where 参数 = '%s' and 时间 between" ("condition"), w333) -> (resulting string=w331:string)  [unwired: 2 in, 1 out]
          n132 = Concatenate Strings(w331, w328, "and" ("字符串"), w324, " order by 时间 asc" ("字符串")) -> (w332:string)
          n133 = call "SQL查询.vi"("condition"=w332, "table输入"=w322, "database"="database3.mdb") -> ("error out"=w320:errorcluster, "data"=w321:string[][])  [unwired: 5 in, 2 out]
        }
      }
    }
    frame "提取仪器参数" {
      w376 = 0 ("索引 (行)")
      n134 = call "数据库加密匹配 (子VI).vi"("输入参数"=w353) -> ("Encoded String"=w356:string)  [unwired: 10 in]
      n135 = global read "断电保存全局.vi" "应用环境"() -> (w354:T3)
      n136 = case shown="\"GB212\", 默认" w354 {
        tunnel: [w384 string[] ["时间", "数据类型", "测量量程", "测量精度", "测量间隔", "消解温度", "消解时长", "空白校准时间", "曲线截距", "曲线斜率", "测量检出限", "测量信号值", "线性相关系数", "二次多项式系数", "标样校准时间"] ("columns输出")] -> w355
        tunnel: w353 -> [w383 _]
        frame "STD" {
          n137 = case shown="\"CODMn\"" w383 {
            tunnel: [string[] ["时间", "数据类型", "测量量程", "测量精度", "测量间隔", "消解温度", "消解时长", "空白校准时间", "曲线截距", "曲线斜率", "测量检出限", "测量信号值", "线性相关系数", "二次多项式系数", "标样校准时间", "量程"] ("columns输出") string[] ["时间", "数据类型", "测量量程", "测量精度", "测量间隔", "消解温度", "消解时长", "空白校准时间", "曲线截距", "曲线斜率", "测量检出限", "测量信号值", "线性相关系数", "二次多项式系数", "标样校准时间", "量程标识"] ("columns输出")] -> w384
            frame "CODMn" {
            }
            frame "", Default {
            }
          }
        }
        frame "GB212", Default {
        }
      }
      n138 = call "数据库加密匹配 (子VI).vi"("输入参数"="N") -> ("Encoded String"=w358:string)  [unwired: 10 in]
      n139 = global read "全局 时间2.vi" "时间2"() -> (w367:string)
      n140 = global read "全局 水样时间.vi" "时间"() -> (w365:string)
      n141 = Format Into String(format string="where 数据类型 = '%s' and 时间 between" ("condition"), w358) -> (resulting string=w359:string)  [unwired: 2 in, 1 out]
      n142 = Format Into String(format string="#%s#" ("初始字符串"), w365) -> (resulting string=w372:string)  [unwired: 2 in, 1 out]
      n143 = Format Into String(format string="#%s#" ("初始字符串"), w367) -> (resulting string=w368:string)  [unwired: 2 in, 1 out]
      n144 = Concatenate Strings(w359, w372, "and" ("字符串"), w368, " order by 时间 desc" ("字符串")) -> (w364:string)
      n145 = call "SQL查询.vi"("condition"=w364, "columns"=w355, "table输入"=w353, "database"="database1.mdb") -> ("error out"=w361:errorcluster, "data"=w362:string[][])  [unwired: 4 in, 2 out]
      n146 = Empty Array?(array=w362) -> (empty?=w363:bool)
      n147 = case shown="真" w363 {
        tunnel: [w388 w404] -> w382
        tunnel: w356 -> [_ w392]
        tunnel: [w389 w390] -> w381
        tunnel: w362 -> [w389 _]
        tunnel: w361 -> [w388 _]
        frame False {
        }
        frame True {
          n148 = global read "全局 时间2.vi" "时间2"() -> (w397:string)
          n149 = global read "全局 水样时间.vi" "时间"() -> (w391:string)
          n150 = Format Into String(format string="where 参数 = '%s' and 时间 between" ("condition"), w392) -> (resulting string=w396:string)  [unwired: 2 in, 1 out]
          n151 = Format Into String(format string="#%s#" ("初始字符串"), w391) -> (resulting string=w402:string)  [unwired: 2 in, 1 out]
          n152 = Format Into String(format string="#%s#" ("初始字符串"), w397) -> (resulting string=w398:string)  [unwired: 2 in, 1 out]
          n153 = Concatenate Strings(w396, w402, "and" ("字符串"), w398, " order by 时间 desc" ("字符串")) -> (w403:string)
          n154 = call "SQL查询.vi"("condition"=w403, "table输入"="仪器参数", "database"="database3.mdb") -> ("error out"=w404:errorcluster, "data"=w390:string[][])  [unwired: 5 in, 2 out]
        }
      }
      n155 = Get Date/Time In Seconds() -> (seconds since 1Jan1904=w378:timestamp)
      n156 = Format Date/Time String(time format string (%c)="%Y/%m/%d %H:%M:%S" ("时间格式字符串(%c)"), seconds (now)=w378) -> (date/time string=w379:string)  [unwired: 1 in]
      n157 = Search and Replace String(input string=w379, search string="." ("搜索字符串")) -> (result string=w375:string)  [unwired: 6 in, 3 out]
      n158 = Replace Array Subset(array=w381, new element=w375, index (row)=w376, index (col)=w376) -> (w374:string[][])
    }
    frame "报警信息", "报警信息存表" {
      # "时间"
      n159 = case shown="\"报警信息\", \"报警信息存表\", \"操作日志\", \"系统状态\"" w411 {
        tunnel: ["database1.mdb" ("database") "database3.mdb" ("database")] -> w422
        frame Default {
        }
        frame "报警信息", "报警信息存表", "操作日志", "系统状态" {
        }
      }
      n160 = case shown="\"环境参数\"" w411 {
        tunnel: [w472 "报警信息" ("table输入")] -> w412
        frame "环境参数" {
          n161 = local read "仪器日志参数"() -> (w472:string)
        }
        frame "报警信息", Default {
        }
      }
      n162 = case shown="\"环境参数\"" w407 {
        tunnel: [" order by 时间 desc" ("字符串") "" ("仪器日志参数")] -> w410
        frame "环境参数" {
        }
        frame "报警信息", Default {
        }
      }
      n163 = case shown="\"报警信息\"" w407 {
        tunnel: [w424 w427] -> w408
        tunnel: [w423 w426] -> w409
        tunnel: w406 -> [_ w428]
        frame "", Default {
          n164 = global read "全局 时间2.vi" "时间2"() -> (w423:string)
          n165 = global read "全局 水样时间.vi" "时间"() -> (w424:string)
        }
        frame "报警信息" {
          n166 = global read "全局 时间2.vi" "报警信息索引"() -> (w425:T4)
          n167 = case shown="\"氟化物\"" w428 {
            tunnel: [w429 w433 w436 w439 w442 w445 w448 w451 w454 w457 w460 w463 w466 w469] -> w426
            tunnel: [w430 w432 w434 w437 w440 w443 w446 w449 w452 w455 w458 w461 w464 w467] -> w427
            tunnel: w425 -> [_ w431 w435 w438 w441 w444 w447 w450 w453 w456 w459 w462 w465 w468]
            frame "假", Default {
              n168 = global read "全局 时间2.vi" "时间2"() -> (w429:string)
              n169 = global read "全局 水样时间.vi" "时间"() -> (w430:string)
            }
            frame "CODMn" {
              n170 = Unbundle By Name(w431) -> ("CODMn报警信息索引起始时间"=w432:string)
              n171 = global read "全局 时间2.vi" "时间2"() -> (w433:string)
            }
            frame "氨氮" {
              n172 = Unbundle By Name(w435) -> ("氨氮报警信息索引起始时间"=w434:string)
              n173 = global read "全局 时间2.vi" "时间2"() -> (w436:string)
            }
            frame "总磷" {
              n174 = Unbundle By Name(w438) -> ("总磷报警信息索引起始时间"=w437:string)
              n175 = global read "全局 时间2.vi" "时间2"() -> (w439:string)
            }
            frame "总氮" {
              n176 = Unbundle By Name(w441) -> ("总氮报警信息索引起始时间"=w440:string)
              n177 = global read "全局 时间2.vi" "时间2"() -> (w442:string)
            }
            frame "CODCr" {
              n178 = Unbundle By Name(w444) -> ("CODCr报警信息索引起始时间"=w443:string)
              n179 = global read "全局 时间2.vi" "时间2"() -> (w445:string)
            }
            frame "DO" {
              n180 = Unbundle By Name(w447) -> ("DO报警信息索引起始时间"=w446:string)
              n181 = global read "全局 时间2.vi" "时间2"() -> (w448:string)
            }
            frame "PH" {
              n182 = Unbundle By Name(w450) -> ("PH报警信息索引起始时间"=w449:string)
              n183 = global read "全局 时间2.vi" "时间2"() -> (w451:string)
            }
            frame "电导率" {
              n184 = Unbundle By Name(w453) -> ("比电导率报警信息索引起始时间"=w452:string)
              n185 = global read "全局 时间2.vi" "时间2"() -> (w454:string)
            }
            frame "水温" {
              n186 = Unbundle By Name(w456) -> ("水温报警信息索引起始时间"=w455:string)
              n187 = global read "全局 时间2.vi" "时间2"() -> (w457:string)
            }
            frame "浊度" {
              n188 = Unbundle By Name(w459) -> ("浊度报警信息索引起始时间"=w458:string)
              n189 = global read "全局 时间2.vi" "时间2"() -> (w460:string)
            }
            frame "叶绿素" {
              n190 = Unbundle By Name(w462) -> ("叶绿素报警信息索引起始时间"=w461:string)
              n191 = global read "全局 时间2.vi" "时间2"() -> (w463:string)
            }
            frame "系统" {
              n192 = Unbundle By Name(w465) -> ("系统报警信息索引起始时间"=w464:string)
              n193 = global read "全局 时间2.vi" "时间2"() -> (w466:string)
            }
            frame "氟化物" {
              n194 = Unbundle By Name(w468) -> ("氟化物报警信息索引起始时间"=w467:string)
              n195 = global read "全局 时间2.vi" "时间2"() -> (w469:string)
            }
          }
        }
      }
      n196 = case shown="\"报警信息\", 默认" w407 {
        tunnel: [w476 w480 "where 时间 between" ("condition")] -> w413
        tunnel: w406 -> [w475 w479 _]
        frame "报警信息", Default {
          n197 = call "数据库加密匹配 (子VI).vi"("输入参数"=w475) -> ("Encoded String"=w474:string)  [unwired: 10 in]
          n198 = Format Into String(format string="where 参数 = '%s' and 时间 between" ("condition"), w474) -> (resulting string=w476:string)  [unwired: 2 in, 1 out]
        }
        frame "环境参数" {
          n199 = call "数据库加密匹配 (子VI).vi"("输入参数"=w479) -> ("Encoded String"=w478:string)  [unwired: 10 in]
          n200 = Format Into String(format string="where 参数 = '%s' and 时间 between" ("condition"), w478) -> (resulting string=w480:string)  [unwired: 2 in, 1 out]
        }
        frame "报警信息存表" {
        }
      }
      n201 = Format Into String(format string="#%s#" ("初始字符串"), w409) -> (resulting string=w414:string)  [unwired: 2 in, 1 out]
      n202 = Format Into String(format string="#%s#" ("初始字符串"), w408) -> (resulting string=w418:string)  [unwired: 2 in, 1 out]
      n203 = Concatenate Strings(w413, w418, "and" ("字符串"), w414, w410) -> (w420:string)
      n204 = call "SQL查询.vi"("condition"=w420, "table输入"=w412, "database"=w422) -> ("error out"=w421:errorcluster, "data"=w419:string[][])  [unwired: 5 in, 2 out]
    }
    frame "提取报警信息" {
      w493 = 0 ("索引 (行)")
      # "时间"
      # "提取仪器状态"
      n205 = call "数据库加密匹配 (子VI).vi"("输入参数"=w496) -> ("Encoded String"=w486:string)  [unwired: 10 in]
      n206 = global read "全局 水样时间.vi" "时间"() -> (w502:string)
      n207 = global read "全局 时间2.vi" "时间2"() -> (w503:string)
      n208 = Format Into String(format string="where 参数 = '%s' and 时间 between" ("condition"), w486) -> (resulting string=w506:string)  [unwired: 2 in, 1 out]
      n209 = Format Into String(format string="#%s#" ("初始字符串"), w502) -> (resulting string=w511:string)  [unwired: 2 in, 1 out]
      n210 = Format Into String(format string="#%s#" ("初始字符串"), w503) -> (resulting string=w507:string)  [unwired: 2 in, 1 out]
      n211 = Concatenate Strings(w506, w511, "and" ("字符串"), w507, " order by 时间 desc" ("仪器日志参数")) -> (w512:string)
      n212 = call "SQL查询.vi"("condition"=w512, "columns"=string[] ["时间", "参数", "故障现象"], "table输入"="报警信息", "database"="database3.mdb") -> ("error out"=w513:errorcluster, "data"=w494:string[][])  [unwired: 4 in, 2 out]
      n213 = Index Array(array=w494, index (row)=w493, index (col)=w493) -> (element=w492:string)
      n214 = call "日期字符串格式至时间格式转换(子VI).vi"("data[0]"=w492) -> ("time stamp"=w490:timestamp)  [unwired: 10 in]
      n215 = Get Date/Time In Seconds() -> (seconds since 1Jan1904=w491:timestamp)
      n216 = Subtract(x=w491, y=w490) -> (x-y=w489:dbl)
      n217 = Format Date/Time String(time format string (%c)="%Y/%m/%d %H:%M:%S" ("时间格式字符串(%c)"), seconds (now)=w491) -> (date/time string=w499:string)  [unwired: 1 in]
      n218 = Greater Or Equal?(x=w489, y=86400.0) -> (x >= y?=w485:bool)
      n219 = Search and Replace String(input string=w499, search string="." ("搜索字符串")) -> (result string=w487:string)  [unwired: 6 in, 3 out]
      n220 = case shown="真" w485 {
        tunnel: [w517 w519] -> w497
        tunnel: w494 -> [w516 w521]
        tunnel: w487 -> [w515 w525]
        tunnel: w486 -> [_ w524]
        frame False {
          w518 = 0 ("索引 (行)")
          n221 = Replace Array Subset(array=w516, new element=w515, index (row)=w518, index (col)=w518) -> (w517:string[][])
        }
        frame True {
          n222 = Build Array(w525, w524, "无告警" ("元素")) -> (w520:string[])
          n223 = Replace Array Subset(array=w521, new element=w520, index (row)=0 ("索引 (行)")) -> (w519:string[][])  [unwired: 1 in]
        }
      }
    }
    frame "环境参数" {
      n224 = call "SQL查询.vi"("condition"=" order by 时间 desc" ("字符串"), "columns"=string[] ["时间", "电压", "室温", "湿度", "GPS经度", "GPS纬度"] ("columns输出 2"), "table输入"=w528, "database"="database1.mdb") -> ("error out"=w532:errorcluster, "columns输出"=w527:string[], "data"=w531:string[][])  [unwired: 4 in, 1 out]
    }
    frame Default {
      # "时间格式转换"
      n225 = local read "待发送数据"() -> (w534:string[][])
      n226 = call "数组时间戳格式化(子VI).vi"("待发送数据输入"=w534) -> ("待发送数据输出"=w533:string[][])  [unwired: 10 in]
    }
    frame "实时数据" {
      (unwired) " order by 时间 desc" ("字符串")
      w541 = "database1.mdb" ("database")
      # "上传本地时间点的实时数据"
      # "上传质控数据（空白测试，跨度核查，核查数据，平行样数据）"
      n227 = global read "全局 实时数据参数.vi" "实时数据参数"() -> (w537:string)
      n228 = case shown="\"空白测试\"" w537 {
        tunnel: [w592 w618 w647 w692] -> w556
        tunnel: w537 -> [w589 w613 _ w689]
        tunnel: [w590 w614 w644 w690] -> w552
        tunnel: w542 -> [_ w617 _ _]
        frame "水样测试" {
          n229 = call "数据库加密匹配 (子VI).vi"("输入参数"=w589) -> ("Encoded String"=w588:string)  [unwired: 10 in]
          n230 = call "数据库加密匹配 (子VI).vi"("输入参数"="N") -> ("Encoded String"=w586:string)  [unwired: 10 in]
          n231 = Get Date/Time In Seconds() -> (seconds since 1Jan1904=w600:timestamp)
          n232 = Format Date/Time String(time format string (%c)="%Y%m%d%H%M%S%3u" ("时间格式字符串(%c)"), seconds (now)=w600) -> (date/time string=w598:string)  [unwired: 1 in]
          n233 = local read "查询元素输入"() -> (w593:string)
          n234 = Replace Substring(2:8 ("长度（子字符串长度）"), 3:10 ("偏移量(0)"), 4:"0000" ("子字符串(\"\")"), 5:w598) -> (1:w594:string)  [unwired: 1 out]
          n235 = case shown="\"CODCr加标回收率\", \"CODMn加标回收率\", \"氨氮加标回收率\", \"总氮加标回收率\", \"总磷加标回收率\"" w593 {
            tunnel: w594 -> [w602 w605 _]
            tunnel: [w601 w606 w607] -> w592
            frame Default {
              n236 = Search and Replace String(input string=w602, search string="." ("搜索字符串")) -> (result string=w603:string)  [unwired: 6 in, 3 out]
              n237 = call "格式时间字符串.vi"("字符串"=w603) -> ("连接的字符串"=w601:string)  [unwired: 10 in]
            }
            frame "CODCr", "CODMn", "累积流量", "总氮", "总磷" {
              n238 = call "实时数据查询用2小时间的数据.vi"("字符串"=w605) -> ("连接的字符串"=w606:string)  [unwired: 10 in]
            }
            frame "CODCr加标回收率", "CODMn加标回收率", "氨氮加标回收率", "总氮加标回收率", "总磷加标回收率" {
              n239 = global read "全局 时间2.vi" "加标回收索引起始时间"() -> (w607:string)
            }
          }
          n240 = Format Into String(format string="where 测量模式 ='%s' and 数据类型 ='%s' and 时间 > " ("格式字符串"), w588, w586) -> (resulting string=w590:string)  [unwired: 2 in, 1 out]
        }
        frame "空白测试" {
          n241 = call "数据库加密匹配 (子VI).vi"("输入参数"=w613) -> ("Encoded String"=w612:string)  [unwired: 10 in]
          n242 = global read "全局 时间2.vi" "零点核查索引"() -> (w616:T5)
          n243 = case shown="\"挥发酚\"" w617 {
            tunnel: [w619 w621 w623 w625 w627 w630 w631 w633 w635 w637 w639] -> w618
            tunnel: w616 -> [w620 w622 w624 w626 w628 w629 w632 w634 w636 w638 _]
            frame "CODMn" {
              n244 = Unbundle By Name(w620) -> ("CODMn零点核查索引起始时间"=w619:string)
            }
            frame "CODCr" {
              n245 = Unbundle By Name(w622) -> ("CODCr零点核查索引起始时间"=w621:string)
            }
            frame "氨氮" {
              n246 = Unbundle By Name(w624) -> ("氨氮零点核查索引起始时间"=w623:string)
            }
            frame "总磷" {
              n247 = Unbundle By Name(w626) -> ("总磷零点核查索引起始时间"=w625:string)
            }
            frame "总氮" {
              n248 = Unbundle By Name(w628) -> ("总氮零点核查索引起始时间"=w627:string)
            }
            frame "亚硝酸盐" {
              n249 = Unbundle By Name(w629) -> ("亚硝酸盐零点核查索引起始时间"=w630:string)
            }
            frame "硫化物" {
              n250 = Unbundle By Name(w632) -> ("硫化物零点核查索引起始时间"=w631:string)
            }
            frame "ORP" {
              n251 = Unbundle By Name(w634) -> ("ORP零点核查索引起始时间"=w633:string)
            }
            frame "氟化物" {
              n252 = Unbundle By Name(w636) -> ("氟化物零点核查索引起始时间"=w635:string)
            }
            frame "挥发酚" {
              n253 = Unbundle By Name(w638) -> ("挥发酚零点核查索引起始时间"=w637:string)
            }
            frame "", Default {
              n254 = global read "全局 时间2.vi" "零点核查索引起始时间"() -> (w639:string)
            }
          }
          n255 = call "数据库加密匹配 (子VI).vi"("输入参数"="零点核查") -> ("Encoded String"=w610:string)  [unwired: 10 in]
          n256 = call "数据库加密匹配 (子VI).vi"("输入参数"="M") -> ("Encoded String"=w608:string)  [unwired: 10 in]
          n257 = Format Into String(format string="where (测量模式 ='%s' or 测量模式 = '%s') and 数据类型 <>'%s' and 时间 > " ("格式字符串"), w612, w610, w608) -> (resulting string=w614:string)  [unwired: 2 in, 1 out]
        }
        frame "核查数据" {
          n258 = global read "全局 时间2.vi" "标样核查索引"() -> (w646:T6)
          n259 = local read "查询元素输入"() -> (w648:string)
          n260 = case shown="\"挥发酚\"" w648 {
            tunnel: [w649 w651 w653 w655 w657 w659 w661 w663 w665 w667 w669 w671 w673 w675 w677 w679 w681 w683 w685] -> w647
            tunnel: w646 -> [w650 w652 w654 w656 w658 w660 w662 w664 w666 w668 w670 w672 w674 w676 w678 w680 w682 w684 _]
            frame "CODMn" {
              n261 = Unbundle By Name(w650) -> ("CODMn标样核查索引起始时间"=w649:string)
            }
            frame "CODCr" {
              n262 = Unbundle By Name(w652) -> ("CODCr标样核查索引起始时间"=w651:string)
            }
            frame "氨氮" {
              n263 = Unbundle By Name(w654) -> ("氨氮标样核查索引起始时间"=w653:string)
            }
            frame "总磷" {
              n264 = Unbundle By Name(w656) -> ("总磷标样核查索引起始时间"=w655:string)
            }
            frame "总氮" {
              n265 = Unbundle By Name(w658) -> ("总氮标样核查索引起始时间"=w657:string)
            }
            frame "DO" {
              n266 = Unbundle By Name(w660) -> ("DO标样核查索引起始时间"=w659:string)
            }
            frame "PH" {
              n267 = Unbundle By Name(w662) -> ("PH标样核查索引起始时间"=w661:string)
            }
            frame "比电导率" {
              n268 = Unbundle By Name(w664) -> ("比电导率标样核查索引起始时间"=w663:string)
            }
            frame "水温" {
              n269 = Unbundle By Name(w666) -> ("水温标样核查索引起始时间"=w665:string)
            }
            frame "浊度" {
              n270 = Unbundle By Name(w668) -> ("浊度标样核查索引起始时间"=w667:string)
            }
            frame "叶绿素a" {
              n271 = Unbundle By Name(w670) -> ("叶绿素a标样核查索引起始时间"=w669:string)
            }
            frame "藻密度" {
              n272 = Unbundle By Name(w672) -> ("藻密度标样核查索引起始时间"=w671:string)
            }
            frame "亚硝酸盐" {
              n273 = Unbundle By Name(w674) -> ("亚硝酸盐标样核查索引起始时间"=w673:string)
            }
            frame "硫化物" {
              n274 = Unbundle By Name(w676) -> ("硫化物标样核查索引起始时间"=w675:string)
            }
            frame "ORP" {
              n275 = Unbundle By Name(w678) -> ("ORP标样核查索引起始时间"=w677:string)
            }
            frame "氟化物" {
              n276 = Unbundle By Name(w680) -> ("氟化物标样核查索引起始时间"=w679:string)
            }
            frame "挥发酚" {
              n277 = Unbundle By Name(w682) -> ("挥发酚标样核查索引起始时间"=w681:string)
            }
            frame "氯化物" {
              n278 = Unbundle By Name(w684) -> ("氯化物标样核查索引起始时间"=w683:string)
            }
            frame "", Default {
              n279 = global read "全局 时间2.vi" "标样核查索引起始时间"() -> (w685:string)
            }
          }
          n280 = call "数据库加密匹配 (子VI).vi"("输入参数"="标样核查" ("实时数据参数")) -> ("Encoded String"=w640:string)  [unwired: 10 in]
          n281 = call "数据库加密匹配 (子VI).vi"("输入参数"="M") -> ("Encoded String"=w642:string)  [unwired: 10 in]
          n282 = Format Into String(format string="where 测量模式 ='%s' and 数据类型 <> '%s' and 时间 > " ("格式字符串"), w640, w642) -> (resulting string=w644:string)  [unwired: 2 in, 1 out]
        }
        frame "跨度核查", Default {
          n283 = call "数据库加密匹配 (子VI).vi"("输入参数"=w689) -> ("Encoded String"=w688:string)  [unwired: 10 in]
          n284 = call "数据库加密匹配 (子VI).vi"("输入参数"="M") -> ("Encoded String"=w686:string)  [unwired: 10 in]
          n285 = global read "全局 时间2.vi" "跨度核查索引"() -> (w694:T7)
          n286 = local read "查询元素输入"() -> (w693:string)
          n287 = case shown="\"挥发酚\"" w693 {
            tunnel: [w695 w697 w699 w701 w703 w706 w707 w709 w711 w713 w715] -> w692
            tunnel: w694 -> [w696 w698 w700 w702 w704 w705 w708 w710 w712 w714 _]
            frame "CODMn" {
              n288 = Unbundle By Name(w696) -> ("CODMn跨度核查索引起始时间"=w695:string)
            }
            frame "CODCr" {
              n289 = Unbundle By Name(w698) -> ("CODCr跨度核查索引起始时间"=w697:string)
            }
            frame "氨氮" {
              n290 = Unbundle By Name(w700) -> ("氨氮跨度核查索引起始时间"=w699:string)
            }
            frame "总磷" {
              n291 = Unbundle By Name(w702) -> ("总磷跨度核查索引起始时间"=w701:string)
            }
            frame "总氮" {
              n292 = Unbundle By Name(w704) -> ("总氮跨度核查索引起始时间"=w703:string)
            }
            frame "亚硝酸盐" {
              n293 = Unbundle By Name(w705) -> ("亚硝酸盐跨度核查索引起始时间"=w706:string)
            }
            frame "硫化物" {
              n294 = Unbundle By Name(w708) -> ("硫化物跨度核查索引起始时间"=w707:string)
            }
            frame "ORP" {
              n295 = Unbundle By Name(w710) -> ("ORP跨度核查索引起始时间"=w709:string)
            }
            frame "氟化物" {
              n296 = Unbundle By Name(w712) -> ("氟化物跨度核查索引起始时间"=w711:string)
            }
            frame "挥发酚" {
              n297 = Unbundle By Name(w714) -> ("挥发酚跨度核查索引起始时间"=w713:string)
            }
            frame "", Default {
              n298 = global read "全局 时间2.vi" "跨度核查索引起始时间"() -> (w715:string)
            }
          }
          n299 = Format Into String(format string="where 测量模式 ='%s' and 数据类型 <> '%s' and 时间 > " ("格式字符串"), w688, w686) -> (resulting string=w690:string)  [unwired: 2 in, 1 out]
        }
      }
      n300 = case shown="\"假\", 默认" w537 {
        tunnel: [string[] ["时间", "测量模式", "数据类型", "检测值", "单位", "数据标识", "标样参考值"] ("columns") string[] ["时间", "测量模式", "数据类型", "检测值", "单位", "数据标识", "标样参考值", "跨度值"] ("columns")] -> w547
        frame "假", Default {
        }
        frame "空白测试", "跨度核查" {
        }
      }
      n301 = global read "断电保存全局.vi" "数据发送延时时间/s"() -> (w546:i32)
      n302 = Get Date/Time In Seconds() -> (seconds since 1Jan1904=w545:timestamp)
      n303 = Subtract(x=w545, y=w546) -> (x-y=w544:timestamp)
      n304 = global read "断电保存全局.vi" "数据组合发送"() -> (w549:bool)
      n305 = Seconds To Date/Time(time stamp (now)=w544) -> (date time rec=w551:T8)  [unwired: 1 in]
      n306 = case shown="真" w549 {
        tunnel: w551 -> [w580 w585]
        tunnel: [w580 w584] -> w550
        frame False {
        }
        frame True {
          n307 = Unbundle By Name(w585) -> ("时"=w583:i32)
          n308 = Subtract(x=w583, y=2) -> (x-y=w581:i32)
          n309 = Bundle By Name(cluster=w585, "时"=w581) -> (w584:T8)
        }
      }
      n310 = Date/Time To Seconds(2:w550) -> (0:w555:timestamp)  [unwired: 1 in]
      n311 = Format Date/Time String(time format string (%c)="%Y/%m/%d %H:%M:%S" ("时间格式字符串(%c)"), seconds (now)=w555) -> (date/time string=w553:string)  [unwired: 1 in]
      n312 = Format Into String(format string="#%s#" ("初始字符串"), w556) -> (resulting string=w561:string)  [unwired: 2 in, 1 out]
      n313 = Format Into String(format string="#%s#" ("初始字符串"), w553) -> (resulting string=w558:string)  [unwired: 2 in, 1 out]
      n314 = Concatenate Strings(w552, w561, "and 时间 < " ("字符串"), w558, " order by 时间 asc" ("字符串")) -> (w540:string)
      n315 = call "SQL查询.vi"("condition"=w540, "columns"=w547, "table输入"=w542, "database"=w541) -> ("error out"=w543:errorcluster, "data"=w539:string[][])  [unwired: 4 in, 2 out]
      n316 = case shown="错误" w543 {
        selector: w543 -> [w562 _]
        tunnel: w537 -> [_ w570]
        tunnel: w542 -> [_ w569]
        tunnel: w541 -> [_ w568]
        tunnel: w540 -> [_ w567]
        tunnel: w539 -> [w563 w565]
        tunnel: [w563 w566] -> w538
        tunnel: [w562 w564] -> w536
        frame No Error {
        }
        frame Error {
          # "兼容旧数据库没有跨度值版本"
          n317 = case shown="\"空白测试\", \"跨度核查\"" w570 {
            tunnel: w569 -> [_ w576]
            tunnel: w568 -> [_ w575]
            tunnel: w567 -> [_ w574]
            tunnel: [w571 w573] -> w566
            tunnel: w565 -> [w571 _]
            tunnel: [_ w572] -> w564
            frame "假", Default {
            }
            frame "空白测试", "跨度核查" {
              n318 = call "SQL查询.vi"("condition"=w574, "columns"=string[] ["时间", "测量模式", "数据类型", "检测值", "单位", "数据标识", "标样参考值"], "table输入"=w576, "database"=w575) -> ("error out"=w572:errorcluster, "data"=w573:string[][])  [unwired: 4 in, 2 out]
            }
          }
        }
      }
      n319 = case shown="默认" w542 {
        tunnel: w542 -> [_ w718]
        tunnel: w540 -> [_ w717]
        tunnel: w538 -> [_ w716]
        frame Default {
        }
        frame "CODCr", "总氮", "总磷" {
          n320 = global write "全局 实时数据参数.vi" "参数"(w718) -> ()
          n321 = global write "全局 实时数据参数.vi" "data"(w716) -> ()
          n322 = global write "全局 实时数据参数.vi" "连接的字符串"(w717) -> ()
        }
      }
    }
    frame "加标回收" {
      w730 = "加标回收率" ("字符串")
      # "上传加标回收数据"
      n323 = call "数据库加密匹配 (子VI).vi"("输入参数"=w720) -> ("Encoded String"=w719:string)  [unwired: 10 in]
      n324 = global read "全局 数据发送重叠.vi" "掉线指示灯"() -> (w731:bool)
      n325 = case shown="假" w731 {
        tunnel: [w746 w762] -> w732
        frame False {
          n326 = global read "全局 时间2.vi" "加标回收索引"() -> (w752:T9)
          n327 = Unbundle By Name(w752) -> ("氨氮加标回收索引起始时间"=w751:string, "总磷加标回收索引起始时间"=w750:string, "总氮加标回收索引起始时间"=w749:string, "CODMn加标回收索引起始时间"=w748:string, "CODCr加标回收索引起始时间"=w747:string, "氟化物加标回收索引起始时间"=w745:string, "挥发酚加标回收索引起始时间"=w744:string)
          n328 = local read "查询元素输入"() -> (w753:string)
          n329 = case shown="\"挥发酚加标回收率\"" w753 {
            tunnel: [w754 w755 w756 w757 w758 w759 w760 w761] -> w746
            tunnel: w751 -> [_ _ w756 _ _ _ _ _]
            tunnel: w750 -> [_ _ _ w757 _ _ _ _]
            tunnel: w749 -> [_ _ _ _ w758 _ _ _]
            tunnel: w748 -> [w754 _ _ _ _ _ _ _]
            tunnel: w747 -> [_ w755 _ _ _ _ _ _]
            tunnel: w745 -> [_ _ _ _ _ w759 _ _]
            tunnel: w744 -> [_ _ _ _ _ _ w760 _]
            frame "CODMn加标回收率" {
            }
            frame "CODCr加标回收率" {
            }
            frame "氨氮加标回收率" {
            }
            frame "总磷加标回收率" {
            }
            frame "总氮加标回收率" {
            }
            frame "氟化物加标回收率" {
            }
            frame "挥发酚加标回收率" {
            }
            frame "", Default {
              n330 = global read "全局 时间2.vi" "加标回收索引起始时间"() -> (w761:string)
            }
          }
        }
        frame True {
          n331 = global read "全局 数据发送重叠.vi" "TCP掉线时间节点"() -> (w762:string)
        }
      }
      n332 = global read "断电保存全局.vi" "数据发送延时时间/s"() -> (w723:i32)
      n333 = Get Date/Time In Seconds() -> (seconds since 1Jan1904=w722:timestamp)
      n334 = Subtract(x=w722, y=w723) -> (x-y=w721:timestamp)
      n335 = Seconds To Date/Time(time stamp (now)=w721) -> (date time rec=w727:T8)  [unwired: 1 in]
      n336 = Date/Time To Seconds(2:w727) -> (0:w729:timestamp)  [unwired: 1 in]
      n337 = Format Date/Time String(time format string (%c)="%Y/%m/%d %H:%M:%S" ("时间格式字符串(%c)"), seconds (now)=w729) -> (date/time string=w726:string)  [unwired: 1 in]
      n338 = Format Into String(format string="#%s#" ("初始字符串"), w732) -> (resulting string=w743:string)  [unwired: 2 in, 1 out]
      n339 = Format Into String(format string="#%s#" ("初始字符串"), w726) -> (resulting string=w739:string)  [unwired: 2 in, 1 out]
      n340 = Concatenate Strings("where 参数 ='" ("condition"), w719, "' and 时间 > ", w743, "and 时间 < " ("字符串"), w739, " order by 时间 asc" ("字符串")) -> (w734:string)
      n341 = call "SQL查询.vi"("condition"=w734, "columns"=string[] ["时间", "参数", "加标前水样测试时间", "加标前水样浓度值", "加标后水样浓度值", "加标母液浓度值", "加标体积", "加标水杯定容体积", "加标回收率"], "table输入"=w730, "database"="database1.mdb") -> ("error out"=w735:errorcluster, "data"=w733:string[][])  [unwired: 4 in, 2 out]
      n342 = case shown="默认" w730 {
        tunnel: w730 -> [_ w765]
        tunnel: w734 -> [_ w764]
        tunnel: w733 -> [_ w763]
        frame Default {
        }
        frame "CODCr", "总氮", "总磷" {
          n343 = global write "全局 实时数据参数.vi" "data"(w763) -> ()
          n344 = global write "全局 实时数据参数.vi" "参数"(w765) -> ()
          n345 = global write "全局 实时数据参数.vi" "连接的字符串"(w764) -> ()
        }
      }
    }
    frame "平行样测试" {
      w777 = "平行样测试" ("字符串")
      # "上传本地时间点的实时数据"
      # "上传平行样数据"
      n346 = call "数据库加密匹配 (子VI).vi"("输入参数"=w767) -> ("Encoded String"=w766:string)  [unwired: 10 in]
      n347 = global read "全局 数据发送重叠.vi" "掉线指示灯"() -> (w778:bool)
      n348 = case shown="假" w778 {
        tunnel: [w803 w812] -> w779
        frame False {
          n349 = global read "全局 时间2.vi" "平行样索引"() -> (w801:T10)
          n350 = Unbundle By Name(w801) -> ("氨氮平行样索引起始时间"=w800:string, "总磷平行样索引起始时间"=w799:string, "总氮平行样索引起始时间"=w798:string, "CODMn平行样索引起始时间"=w797:string, "CODCr平行样索引起始时间"=w796:string, "氟化物平行样索引起始时间"=w795:string, "挥发酚平行样索引起始时间"=w794:string)
          n351 = local read "查询元素输入"() -> (w802:string)
          n352 = case shown="\"挥发酚\"" w802 {
            tunnel: [w804 w805 w806 w807 w808 w809 w810 w811] -> w803
            tunnel: w800 -> [_ _ w806 _ _ _ _ _]
            tunnel: w799 -> [_ _ _ w807 _ _ _ _]
            tunnel: w798 -> [_ _ _ _ w808 _ _ _]
            tunnel: w797 -> [w804 _ _ _ _ _ _ _]
            tunnel: w796 -> [_ w805 _ _ _ _ _ _]
            tunnel: w795 -> [_ _ _ _ _ w809 _ _]
            tunnel: w794 -> [_ _ _ _ _ _ w810 _]
            frame "CODMn" {
            }
            frame "CODCr" {
            }
            frame "氨氮" {
            }
            frame "总磷" {
            }
            frame "总氮" {
            }
            frame "氟化物" {
            }
            frame "挥发酚" {
            }
            frame "", Default {
              n353 = global read "全局 时间2.vi" "平行样索引起始时间"() -> (w811:string)
            }
          }
        }
        frame True {
          n354 = global read "全局 数据发送重叠.vi" "TCP掉线时间节点"() -> (w812:string)
        }
      }
      n355 = global read "断电保存全局.vi" "数据发送延时时间/s"() -> (w770:i32)
      n356 = Get Date/Time In Seconds() -> (seconds since 1Jan1904=w769:timestamp)
      n357 = Subtract(x=w769, y=w770) -> (x-y=w768:timestamp)
      n358 = Seconds To Date/Time(time stamp (now)=w768) -> (date time rec=w774:T8)  [unwired: 1 in]
      n359 = Date/Time To Seconds(2:w774) -> (0:w776:timestamp)  [unwired: 1 in]
      n360 = Format Date/Time String(time format string (%c)="%Y/%m/%d %H:%M:%S" ("时间格式字符串(%c)"), seconds (now)=w776) -> (date/time string=w773:string)  [unwired: 1 in]
      n361 = Format Into String(format string="#%s#" ("初始字符串"), w779) -> (resulting string=w793:string)  [unwired: 2 in, 1 out]
      n362 = Format Into String(format string="#%s#" ("初始字符串"), w773) -> (resulting string=w789:string)  [unwired: 2 in, 1 out]
      n363 = Concatenate Strings("where 参数 ='" ("condition"), w766, "' and 时间 > ", w793, "and 时间 < " ("字符串"), w789, " order by 时间 asc" ("字符串")) -> (w781:string)
      n364 = call "SQL查询.vi"("condition"=w781, "columns"=string[] ["时间", "参数", "第一次水样浓度值", "第二次水样测试时间", "第二次水样浓度值"], "table输入"=w777, "database"="database1.mdb") -> ("error out"=w783:errorcluster, "data"=w780:string[][])  [unwired: 4 in, 2 out]
      n365 = case shown="默认" w777 {
        tunnel: w777 -> [_ w815]
        tunnel: w781 -> [_ w814]
        tunnel: w780 -> [_ w813]
        frame Default {
        }
        frame "CODCr", "总氮", "总磷" {
          n366 = global write "全局 实时数据参数.vi" "data"(w813) -> ()
          n367 = global write "全局 实时数据参数.vi" "参数"(w815) -> ()
          n368 = global write "全局 实时数据参数.vi" "连接的字符串"(w814) -> ()
        }
      }
      n369 = case shown="假" FALSE {
        tunnel: [w817 w820] -> w785
        tunnel: w780 -> [w817 w819]
        tunnel: w783 -> [w816 w818]
        tunnel: [w816 w818] -> w782
        frame False {
        }
        frame True {
          # "数字字符串精度转换保留"
          n370 = Index Array(array=w819, index (col)=3 ("禁用的索引 (列)")) -> (element=w826:string[])  [unwired: 1 in]
          n371 = for {
            tunnel: w826 -> [w829] mode=indexing
            tunnel: [w828] -> w822 mode=indexing
            n372 = Fract/Exp String To Number(string=w829) -> (number=w830:dbl)  [unwired: 3 in, 1 out]
            n373 = Number To Fractional String(number=w830, precision (6)=i16 2 ("精度(6)")) -> (F-format string=w828:string)  [unwired: 2 in]
          }
          n374 = Delete From Array(array=w819, length=1 ("长度"), index (col)=3 ("禁用的索引 (列)")) -> (array with subset deleted=w823:string[][])  [unwired: 1 in, 1 out]
          n375 = Insert Into Array(array=w823, index (col)=3 ("禁用的索引 (列)"), new element=w822) -> (w820:string[][])  [unwired: 1 in]
        }
      }
    }
    frame "集成干预测试" {
      # "上传本地时间点的实时数据"
      # "上传集成干预数据"
      n376 = global read "全局 数据发送重叠.vi" "掉线指示灯"() -> (w845:bool)
      n377 = case shown="假" w845 {
        tunnel: [w869 w907] -> w846
        frame False {
          n378 = global read "全局 时间2.vi" "集成干预索引"() -> (w871:T11)
          n379 = local read "查询元素输入"() -> (w870:string)
          n380 = case shown="\"总磷\"" w870 {
            tunnel: [w872 w874 w876 w878 w880 w882 w884 w886 w888 w890 w892 w894 w896 w898 w900 w902 w904 w906] -> w869
            tunnel: w871 -> [w873 w875 w877 w879 w881 w883 w885 w887 w889 w891 w893 w895 w897 w899 w901 w903 w905 _]
            frame "CODMn" {
              n381 = Unbundle By Name(w873) -> ("CODMn集成干预索引起始时间"=w872:string)
            }
            frame "CODCr" {
              n382 = Unbundle By Name(w875) -> ("CODCr集成干预索引起始时间"=w874:string)
            }
            frame "氨氮" {
              n383 = Unbundle By Name(w877) -> ("氨氮集成干预索引起始时间"=w876:string)
            }
            frame "总磷" {
              n384 = Unbundle By Name(w879) -> ("总磷集成干预索引起始时间"=w878:string)
            }
            frame "总氮" {
              n385 = Unbundle By Name(w881) -> ("总氮集成干预索引起始时间"=w880:string)
            }
            frame "DO" {
              n386 = Unbundle By Name(w883) -> ("DO集成干预索引起始时间"=w882:string)
            }
            frame "PH" {
              n387 = Unbundle By Name(w885) -> ("PH集成干预索引起始时间"=w884:string)
            }
            frame "比电导率" {
              n388 = Unbundle By Name(w887) -> ("比电导率集成干预索引起始时间"=w886:string)
            }
            frame "水温" {
              n389 = Unbundle By Name(w889) -> ("水温集成干预索引起始时间"=w888:string)
            }
            frame "浊度" {
              n390 = Unbundle By Name(w891) -> ("浊度集成干预索引起始时间"=w890:string)
            }
            frame "叶绿素a" {
              n391 = Unbundle By Name(w893) -> ("叶绿素a集成干预索引起始时间"=w892:string)
            }
            frame "藻密度" {
              n392 = Unbundle By Name(w895) -> ("藻密度集成干预索引起始时间"=w894:string)
            }
            frame "亚硝酸盐" {
              n393 = Unbundle By Name(w897) -> ("亚硝酸盐集成干预索引起始时间"=w896:string)
            }
            frame "硫化物" {
              n394 = Unbundle By Name(w899) -> ("硫化物集成干预索引起始时间"=w898:string)
            }
            frame "ORP" {
              n395 = Unbundle By Name(w901) -> ("ORP集成干预索引起始时间"=w900:string)
            }
            frame "氟化物" {
              n396 = Unbundle By Name(w903) -> ("氟化物集成干预索引起始时间"=w902:string)
            }
            frame "挥发酚" {
              n397 = Unbundle By Name(w905) -> ("挥发酚集成干预索引起始时间"=w904:string)
            }
            frame "", Default {
              n398 = global read "全局 时间2.vi" "平行样索引起始时间"() -> (w906:string)
            }
          }
        }
        frame True {
          n399 = global read "全局 数据发送重叠.vi" "TCP掉线时间节点"() -> (w907:string)
        }
      }
      n400 = global read "断电保存全局.vi" "应用环境"() -> (w836:T3)
      n401 = case shown="\"STD\"" w836 {
        tunnel: w835 -> [w858 w868]
        tunnel: ["集成干预测试" ("字符串") w868] -> w834
        tunnel: [string[] ["时间", "参数", "集成干预测试浓度值", "集成干预前测试时间", "集成干预前测试浓度值"] ("columns") string[] ["时间", "测量模式", "数据类型", "检测值", "单位", "数据标识", "因子编码", "标样参考值"] ("columns")] -> w833
        tunnel: [w860 w867] -> w832
        frame "STD" {
          n402 = call "数据库加密匹配 (子VI).vi"("输入参数"=w858) -> ("Encoded String"=w857:string)  [unwired: 10 in]
          n403 = Concatenate Strings("where 参数 ='" ("condition"), w857) -> (w860:string)
        }
        frame "GB212", Default {
          n404 = call "数据库加密匹配 (子VI).vi"("输入参数"="集成干预测试" ("字符串")) -> ("Encoded String"=w863:string)  [unwired: 10 in]
          n405 = Concatenate Strings("where 测量模式 ='" ("condition"), w863) -> (w867:string)
        }
      }
      n406 = global read "断电保存全局.vi" "数据发送延时时间/s"() -> (w839:i32)
      n407 = Get Date/Time In Seconds() -> (seconds since 1Jan1904=w838:timestamp)
      n408 = Subtract(x=w838, y=w839) -> (x-y=w837:timestamp)
      n409 = Seconds To Date/Time(time stamp (now)=w837) -> (date time rec=w842:T8)  [unwired: 1 in]
      n410 = Date/Time To Seconds(2:w842) -> (0:w844:timestamp)  [unwired: 1 in]
      n411 = Format Date/Time String(time format string (%c)="%Y/%m/%d %H:%M:%S" ("时间格式字符串(%c)"), seconds (now)=w844) -> (date/time string=w841:string)  [unwired: 1 in]
      n412 = Format Into String(format string="#%s#" ("初始字符串"), w846) -> (resulting string=w856:string)  [unwired: 2 in, 1 out]
      n413 = Format Into String(format string="#%s#" ("初始字符串"), w841) -> (resulting string=w852:string)  [unwired: 2 in, 1 out]
      n414 = Concatenate Strings(w832, "' and 时间 > ", w856, "and 时间 < " ("字符串"), w852, " order by 时间 asc" ("字符串")) -> (w848:string)
      n415 = call "SQL查询.vi"("condition"=w848, "columns"=w833, "table输入"=w834, "database"="database1.mdb") -> ("error out"=w849:errorcluster, "data"=w847:string[][])  [unwired: 4 in, 2 out]
      n416 = case shown="\"CODCr\", \"总氮\", \"总磷\"" w834 {
        tunnel: w834 -> [_ w910]
        tunnel: w848 -> [_ w909]
        tunnel: w847 -> [_ w908]
        frame Default {
        }
        frame "CODCr", "总氮", "总磷" {
          n417 = global write "全局 实时数据参数.vi" "参数"(w910) -> ()
          n418 = global write "全局 实时数据参数.vi" "data"(w908) -> ()
          n419 = global write "全局 实时数据参数.vi" "连接的字符串"(w909) -> ()
        }
      }
    }
    frame "提取加标回收" {
      w915 = "加标回收率" ("字符串")
      # "上传本地时间点的实时数据"
      n420 = call "数据库加密匹配 (子VI).vi"("输入参数"=w912) -> ("Encoded String"=w911:string)  [unwired: 10 in]
      n421 = global read "全局 数据发送重叠.vi" "掉线指示灯"() -> (w916:bool)
      n422 = case shown="假" w916 {
        tunnel: [w932 w933] -> w917
        frame False {
          n423 = global read "起始时间.vi" "起始时间"() -> (w932:string)
        }
        frame True {
          n424 = global read "全局 数据发送重叠.vi" "TCP掉线时间节点"() -> (w933:string)
        }
      }
      n425 = global read "起始时间.vi" "结束时间"() -> (w914:string)
      n426 = Format Into String(format string="#%s#" ("初始字符串"), w917) -> (resulting string=w931:string)  [unwired: 2 in, 1 out]
      n427 = Format Into String(format string="#%s#" ("初始字符串"), w914) -> (resulting string=w927:string)  [unwired: 2 in, 1 out]
      n428 = Concatenate Strings("where 参数 ='" ("condition"), w911, "' and 时间 between ", w931, "and" ("字符串"), w927) -> (w919:string)
      n429 = call "SQL查询.vi"("condition"=w919, "columns"=string[] ["时间", "参数", "加标前水样测试时间", "加标前水样浓度值", "加标后水样浓度值", "加标母液浓度值", "加标体积", "加标水杯定容体积", "加标回收率"], "table输入"=w915, "database"="database1.mdb") -> ("error out"=w921:errorcluster, "data"=w918:string[][])  [unwired: 4 in, 2 out]
      n430 = case shown="\"CODCr\", \"总氮\", \"总磷\"" w915 {
        tunnel: w915 -> [_ w936]
        tunnel: w919 -> [_ w935]
        tunnel: w918 -> [_ w934]
        frame Default {
        }
        frame "CODCr", "总氮", "总磷" {
          n431 = global write "全局 实时数据参数.vi" "data"(w934) -> ()
          n432 = global write "全局 实时数据参数.vi" "参数"(w936) -> ()
          n433 = global write "全局 实时数据参数.vi" "连接的字符串"(w935) -> ()
        }
      }
      n434 = case shown="假" FALSE {
        tunnel: [w938 w941] -> w923
        tunnel: w918 -> [w938 w940]
        tunnel: w921 -> [w937 w939]
        tunnel: [w937 w939] -> w920
        frame False {
        }
        frame True {
          # "数字字符串精度转换保留"
          n435 = Index Array(array=w940, index (col)=3 ("禁用的索引 (列)")) -> (element=w947:string[])  [unwired: 1 in]
          n436 = for {
            tunnel: w947 -> [w950] mode=indexing
            tunnel: [w949] -> w943 mode=indexing
            n437 = Fract/Exp String To Number(string=w950) -> (number=w951:dbl)  [unwired: 3 in, 1 out]
            n438 = Number To Fractional String(number=w951, precision (6)=i16 2 ("精度(6)")) -> (F-format string=w949:string)  [unwired: 2 in]
          }
          n439 = Delete From Array(array=w940, length=1 ("长度"), index (col)=3 ("禁用的索引 (列)")) -> (array with subset deleted=w944:string[][])  [unwired: 1 in, 1 out]
          n440 = Insert Into Array(array=w944, index (col)=3 ("禁用的索引 (列)"), new element=w943) -> (w941:string[][])  [unwired: 1 in]
        }
      }
    }
    frame "提取平行样" {
      w957 = "平行样测试" ("字符串")
      # "上传本地时间点的实时数据"
      n441 = call "数据库加密匹配 (子VI).vi"("输入参数"=w954) -> ("Encoded String"=w953:string)  [unwired: 10 in]
      n442 = global read "全局 数据发送重叠.vi" "掉线指示灯"() -> (w958:bool)
      n443 = case shown="假" w958 {
        tunnel: [w974 w975] -> w959
        frame False {
          n444 = global read "起始时间.vi" "起始时间"() -> (w974:string)
        }
        frame True {
          n445 = global read "全局 数据发送重叠.vi" "TCP掉线时间节点"() -> (w975:string)
        }
      }
      n446 = global read "起始时间.vi" "结束时间"() -> (w956:string)
      n447 = Format Into String(format string="#%s#" ("初始字符串"), w959) -> (resulting string=w973:string)  [unwired: 2 in, 1 out]
      n448 = Format Into String(format string="#%s#" ("初始字符串"), w956) -> (resulting string=w969:string)  [unwired: 2 in, 1 out]
      n449 = Concatenate Strings("where 参数 ='" ("condition"), w953, "' and 时间 between ", w973, "and" ("字符串"), w969) -> (w961:string)
      n450 = call "SQL查询.vi"("condition"=w961, "columns"=string[] ["时间", "参数", "第一次水样浓度值", "第二次水样测试时间", "第二次水样浓度值"], "table输入"=w957, "database"="database1.mdb") -> ("error out"=w963:errorcluster, "data"=w960:string[][])  [unwired: 4 in, 2 out]
      n451 = case shown="\"CODCr\", \"总氮\", \"总磷\"" w957 {
        tunnel: w957 -> [_ w978]
        tunnel: w961 -> [_ w977]
        tunnel: w960 -> [_ w976]
        frame Default {
        }
        frame "CODCr", "总氮", "总磷" {
          n452 = global write "全局 实时数据参数.vi" "data"(w976) -> ()
          n453 = global write "全局 实时数据参数.vi" "参数"(w978) -> ()
          n454 = global write "全局 实时数据参数.vi" "连接的字符串"(w977) -> ()
        }
      }
      n455 = case shown="假" FALSE {
        tunnel: [w980 w983] -> w965
        tunnel: w960 -> [w980 w982]
        tunnel: w963 -> [w979 w981]
        tunnel: [w979 w981] -> w962
        frame False {
        }
        frame True {
          # "数字字符串精度转换保留"
          n456 = Index Array(array=w982, index (col)=3 ("禁用的索引 (列)")) -> (element=w989:string[])  [unwired: 1 in]
          n457 = for {
            tunnel: w989 -> [w992] mode=indexing
            tunnel: [w991] -> w985 mode=indexing
            n458 = Fract/Exp String To Number(string=w992) -> (number=w993:dbl)  [unwired: 3 in, 1 out]
            n459 = Number To Fractional String(number=w993, precision (6)=i16 2 ("精度(6)")) -> (F-format string=w991:string)  [unwired: 2 in]
          }
          n460 = Delete From Array(array=w982, length=1 ("长度"), index (col)=3 ("禁用的索引 (列)")) -> (array with subset deleted=w986:string[][])  [unwired: 1 in, 1 out]
          n461 = Insert Into Array(array=w986, index (col)=3 ("禁用的索引 (列)"), new element=w985) -> (w983:string[][])  [unwired: 1 in]
        }
      }
    }
    frame "提取集成干预" {
      # "上传本地时间点的实时数据"
      n462 = global read "断电保存全局.vi" "应用环境"() -> (w999:T3)
      n463 = case shown="\"GB212\", 默认" w999 {
        tunnel: w995 -> [w1017 w1027]
        tunnel: ["集成干预测试" ("字符串") w1027] -> w997
        tunnel: [string[] ["时间", "参数", "集成干预测试浓度值", "集成干预前测试时间", "集成干预前测试浓度值"] ("columns") string[] ["时间", "测量模式", "数据类型", "检测值", "单位", "数据标识", "因子编码", "标样参考值"] ("columns")] -> w998
        tunnel: [w1019 w1026] -> w996
        frame "STD" {
          n464 = call "数据库加密匹配 (子VI).vi"("输入参数"=w1017) -> ("Encoded String"=w1016:string)  [unwired: 10 in]
          n465 = Concatenate Strings("where 参数 ='" ("condition"), w1016) -> (w1019:string)
        }
        frame "GB212", Default {
          n466 = call "数据库加密匹配 (子VI).vi"("输入参数"="集成干预测试" ("字符串")) -> ("Encoded String"=w1022:string)  [unwired: 10 in]
          n467 = Concatenate Strings("where 测量模式 ='" ("condition"), w1022) -> (w1026:string)
        }
      }
      n468 = global read "全局 数据发送重叠.vi" "掉线指示灯"() -> (w1001:bool)
      n469 = case shown="假" w1001 {
        tunnel: [w1028 w1029] -> w1002
        frame False {
          n470 = global read "起始时间.vi" "起始时间"() -> (w1028:string)
        }
        frame True {
          n471 = global read "全局 数据发送重叠.vi" "TCP掉线时间节点"() -> (w1029:string)
        }
      }
      n472 = global read "起始时间.vi" "结束时间"() -> (w1000:string)
      n473 = Format Into String(format string="#%s#" ("初始字符串"), w1002) -> (resulting string=w1015:string)  [unwired: 2 in, 1 out]
      n474 = Format Into String(format string="#%s#" ("初始字符串"), w1000) -> (resulting string=w1011:string)  [unwired: 2 in, 1 out]
      n475 = Concatenate Strings(w996, "' and 时间 between ", w1015, "and" ("字符串"), w1011) -> (w1004:string)
      n476 = call "SQL查询.vi"("condition"=w1004, "columns"=w998, "table输入"=w997, "database"="database1.mdb") -> ("error out"=w1006:errorcluster, "data"=w1003:string[][])  [unwired: 4 in, 2 out]
      n477 = case shown="\"CODCr\", \"总氮\", \"总磷\"" w997 {
        tunnel: w997 -> [_ w1032]
        tunnel: w1004 -> [_ w1031]
        tunnel: w1003 -> [_ w1030]
        frame Default {
        }
        frame "CODCr", "总氮", "总磷" {
          n478 = global write "全局 实时数据参数.vi" "data"(w1030) -> ()
          n479 = global write "全局 实时数据参数.vi" "参数"(w1032) -> ()
          n480 = global write "全局 实时数据参数.vi" "连接的字符串"(w1031) -> ()
        }
      }
      n481 = case shown="假" FALSE {
        tunnel: [w1034 w1037] -> w1008
        tunnel: w1003 -> [w1034 w1036]
        tunnel: w1006 -> [w1033 w1035]
        tunnel: [w1033 w1035] -> w1005
        frame False {
        }
        frame True {
          # "数字字符串精度转换保留"
          n482 = Index Array(array=w1036, index (col)=3 ("禁用的索引 (列)")) -> (element=w1043:string[])  [unwired: 1 in]
          n483 = for {
            tunnel: w1043 -> [w1046] mode=indexing
            tunnel: [w1045] -> w1039 mode=indexing
            n484 = Fract/Exp String To Number(string=w1046) -> (number=w1047:dbl)  [unwired: 3 in, 1 out]
            n485 = Number To Fractional String(number=w1047, precision (6)=i16 2 ("精度(6)")) -> (F-format string=w1045:string)  [unwired: 2 in]
          }
          n486 = Delete From Array(array=w1036, length=1 ("长度"), index (col)=3 ("禁用的索引 (列)")) -> (array with subset deleted=w1040:string[][])  [unwired: 1 in, 1 out]
          n487 = Insert Into Array(array=w1040, index (col)=3 ("禁用的索引 (列)"), new element=w1039) -> (w1037:string[][])  [unwired: 1 in]
        }
      }
    }
    frame "提取实时数据" {
      # "上传给定时间段之间的实时数据"
      n488 = global read "全局 实时数据参数.vi" "实时数据参数"() -> (w1050:string)
      n489 = call "数据库加密匹配 (子VI).vi"("输入参数"=w1050) -> ("Encoded String"=w1049:string)  [unwired: 10 in]
      n490 = global read "起始时间.vi" "起始时间"() -> (w1061:string)
      n491 = global read "起始时间.vi" "结束时间"() -> (w1060:string)
      n492 = Format Into String(format string="#%s#" ("初始字符串"), w1061) -> (resulting string=w1068:string)  [unwired: 2 in, 1 out]
      n493 = Format Into String(format string="#%s#" ("初始字符串"), w1060) -> (resulting string=w1062:string)  [unwired: 2 in, 1 out]
      n494 = Concatenate Strings("where 测量模式 ='" ("condition"), w1049, "' and 时间 between ", w1068, "and" ("字符串"), w1062) -> (w1066:string)
      n495 = call "SQL查询.vi"("condition"=w1066, "columns"=string[] ["时间", "测量模式", "数据类型", "检测值", "单位", "数据标识", "标样参考值"], "table输入"=w1052, "database"="database1.mdb") -> ("error out"=w1057:errorcluster, "data"=w1059:string[][])  [unwired: 4 in, 2 out]
      n496 = case shown="假" FALSE {
        tunnel: w1059 -> [w1070 w1078]
        tunnel: [w1070 w1072] -> w1058
        tunnel: w1057 -> [w1069 w1071]
        tunnel: [w1069 w1071] -> w1056
        frame False {
        }
        frame True {
          # "数字字符串精度转换保留"
          n497 = Index Array(array=w1078, index (col)=3 ("禁用的索引 (列)")) -> (element=w1079:string[])  [unwired: 1 in]
          n498 = for {
            tunnel: w1079 -> [w1082] mode=indexing
            tunnel: [w1081] -> w1074 mode=indexing
            n499 = Fract/Exp String To Number(string=w1082) -> (number=w1083:dbl)  [unwired: 3 in, 1 out]
            n500 = Number To Fractional String(number=w1083, precision (6)=i16 2 ("精度(6)")) -> (F-format string=w1081:string)  [unwired: 2 in]
          }
          n501 = Delete From Array(array=w1078, length=1 ("长度"), index (col)=3 ("禁用的索引 (列)")) -> (array with subset deleted=w1075:string[][])  [unwired: 1 in, 1 out]
          n502 = Insert Into Array(array=w1075, index (col)=3 ("禁用的索引 (列)"), new element=w1074) -> (w1072:string[][])  [unwired: 1 in]
        }
      }
    }
  }
  "待发送数据" <- w1
  "columns输出" <- w2
  n503 = call <vilib>:"Clear Errors.vi"("error in (no error)"=w8) -> ("error out"=→"error out":errorcluster)  [unwired: 5 in, 1 out]
  n504 = Index Array(array=w1, index (row)=0 ("索引 (行)")) -> (element=→"待发送第一条数据":string[])  [unwired: 1 in]
